vi "svx_Timebase Facade.vi"(0 "Data In":T8, 2 "Display State In":T3={"X Scale"={"Name"="Time", "FString"="%#.2g", "Major Color"=16777238, "Minor Color"=16777216, "Grid Style"=1, "Maximum"=0.5, "Minimum"=0.0, "Autoscale"=TRUE, "Show Scale Label"={"Probe X"=FALSE, "Probe Y"=TRUE}, "Show Scale"={"Probe X"=TRUE, "Probe Y"=TRUE}, "Autoscale Once"=FALSE}, "Y Scale"={"Name"="Amplitude", "FString"="%#.2g", "Major Color"=16777238, "Minor Color"=16777216, "Scale Visible"=TRUE, " Label Visible"=TRUE, "Grid Style"=1, "Autoscale"=TRUE, "Maximum"={"Probe X"=1.0, "Probe Y"=1.0}, "Minimum"={"Probe X"=-1.0, "Probe Y"=-1.0}, "Autoscale Once"=FALSE}, "Plot"={"Point Style"=0, "Line Width"=0, "Line Style"=0, "Plot Color"=16860, "Point/fill"=16860}, "Tacho Point Color"=16711680, "Property Name"=[], "Container Bounds"={"Width"=640, "Height"=360}, "Background color"=16777226, "Legend Visible"=TRUE, "Scale Range Change"=refnum, "Strings[]"={"Custom pair name"=FALSE, "Row Strings []"=[], "Column Strings []"=[]}, "Cursor"={"Cursor Point Style"=13, "Cursor Style"=5, "Cursor Line Width"=1, "Cursor Line Style"=0, "Cursor Color"=16860, "Cursor Name Visible"=TRUE, "Cursor Visible"=TRUE, "Cursor Lock"=FALSE, "Cursor Index"=0}, "Index"=[], "Legend Width"=200, " Parents Tags"=[], "Children Tags"=[], "Open?"=[], "Label"="Timebase Plot", "Cursor X Pos"={"X"=0.0, "Y"=0.0}, "Cursor Y Pos"={"X"=0.0, "Y"=0.0}, "Graph Type"=enum."Probe X and Y", "Prev Graph Type"=enum."Probe X and Y", "Prev Legend Visible"=TRUE, "Cursor Release"=refnum, "Pair Strings Changed?"=FALSE, "Cursor ID"=refnum, "Legend Background"=16777226, "Legend Font"=16777222, "Probe Y Label"="Probe Y", "Probe X Label"="Probe X", "Probe X Label Visible"=TRUE, "Probe Y Label Visible"=TRUE, "Tree Item Width"=200, "# Custom RowStr"=0, "# Custom ColStr"=0, "Property Name"=refnum, "Data Related State"=refnum}, 3 "Container State":T7) -> (6 "Data Out":T8, 7 "Display State Out":T3={"X Scale"={"Name"="Time", "FString"="%#.2g", "Major Color"=16777238, "Minor Color"=16777216, "Grid Style"=1, "Maximum"=0.5, "Minimum"=0.0, "Autoscale"=TRUE, "Show Scale Label"={"Probe X"=FALSE, "Probe Y"=TRUE}, "Show Scale"={"Probe X"=TRUE, "Probe Y"=TRUE}, "Autoscale Once"=FALSE}, "Y Scale"={"Name"="Amplitude", "FString"="%#.2g", "Major Color"=16777238, "Minor Color"=16777216, "Scale Visible"=TRUE, " Label Visible"=TRUE, "Grid Style"=1, "Autoscale"=TRUE, "Maximum"={"Probe X"=1.0, "Probe Y"=1.0}, "Minimum"={"Probe X"=-1.0, "Probe Y"=-1.0}, "Autoscale Once"=FALSE}, "Plot"={"Point Style"=0, "Line Width"=0, "Line Style"=0, "Plot Color"=16860, "Point/fill"=16860}, "Tacho Point Color"=16711680, "Property Name"=[], "Container Bounds"={"Width"=640, "Height"=360}, "Background color"=16777226, "Legend Visible"=TRUE, "Scale Range Change"=refnum, "Strings[]"={"Custom pair name"=FALSE, "Row Strings []"=[], "Column Strings []"=[]}, "Cursor"={"Cursor Point Style"=13, "Cursor Style"=5, "Cursor Line Width"=1, "Cursor Line Style"=0, "Cursor Color"=16860, "Cursor Name Visible"=TRUE, "Cursor Visible"=TRUE, "Cursor Lock"=FALSE, "Cursor Index"=0}, "Index"=[], "Legend Width"=200, " Parents Tags"=[], "Children Tags"=[], "Open?"=[], "Label"="Timebase Plot", "Cursor X Pos"={"X"=0.0, "Y"=0.0}, "Cursor Y Pos"={"X"=0.0, "Y"=0.0}, "Graph Type"=enum."Probe X and Y", "Prev Graph Type"=enum."Probe X and Y", "Prev Legend Visible"=TRUE, "Cursor Release"=refnum, "Pair Strings Changed?"=FALSE, "Cursor ID"=refnum, "Legend Background"=16777226, "Legend Font"=16777222, "Probe Y Label"="Probe Y", "Probe X Label"="Probe X", "Probe X Label Visible"=TRUE, "Probe Y Label Visible"=TRUE, "Tree Item Width"=200, "# Custom RowStr"=0, "# Custom ColStr"=0, "Property Name"=refnum, "Data Related State"=refnum}, 8 "Action":T2)   [LabVIEW 2017, in "SVX Timebase.xctl"]
uses:
  <vilib>/addons/_XControls/Timebase Plot/SVX Timebase.xctl
  <vilib>/addons/_XControls/Timebase Plot/subVIs/svx_Timebase Data.ctl
  <vilib>/_xctls/Container State.ctl
  <vilib>/addons/_XControls/Timebase Plot/subVIs/svx_Timebase State.ctl
  <vilib>/addons/_XControls/Timebase Plot/subVIs/svx_Timebase Bounds.ctl
  <vilib>/addons/_XControls/Timebase Plot/subVIs/svx_Timebase Graph Types.ctl
  <vilib>/addons/_XControls/Timebase Plot/subVIs/svx_Timebase Data Related State.ctl
  <vilib>/_xctls/Action.ctl
  <vilib>/Utility/miscctls.llb/LVPoint32TypeDef.ctl
  <vilib>/addons/_XControls/Timebase Plot/subVIs/svx_Timebase Core States.ctl
  <vilib>/Utility/cursorutil.llb/Set Cursor (Icon Pict).vi
  <vilib>/Utility/cursorutil.llb/Set Cursor (Cursor ID).vi
  <vilib>/_xctls/XControlSupport.lvlib
panel:
  out "Coords":T1
  out "Orig Legend Width":u32
  out "Orig Coord":i32
  in  "Split":bool
  out "cursor X info":string
  out "cursor Y info":string
  out "Probe Y":T9(graph)=[{"orbit plot X"=[1.0], "orbit plot Y"=[2.0]}, {"orbit plot X"=[2.0], "orbit plot Y"=[4.0]}]
  out "Probe X":T9(graph)=[{"orbit plot X"=[1.0], "orbit plot Y"=[2.0]}, {"orbit plot X"=[2.0], "orbit plot Y"=[4.0]}]
  in  "Tree":string(tree)="Order 3.00"
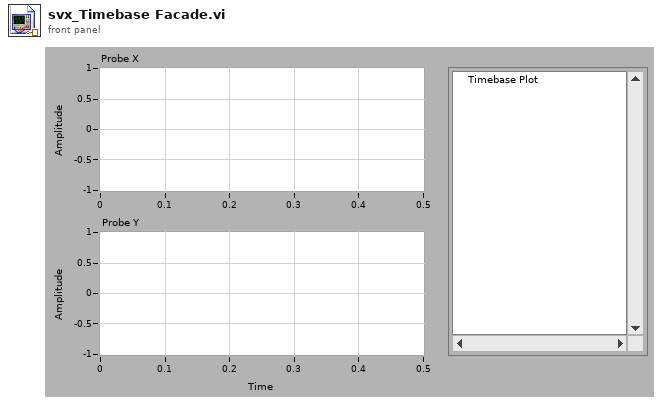
[diagram p1: front panel]
types:
  T1 = typedef "LVPoint32TypeDef.ctl" = cluster{"Horizontal":i32, "Vertical":i32}
  T2 = typedef "XControlSupport.lvlib/Action.ctl" = cluster{"Data Changed?":bool, "State Changed?":bool, "Action Name":string}
  T3 = typedef "SVX Timebase.xctl/svx_Timebase State.ctl" = cluster{"X Scale":cluster{"Name":string, "FString":string, "Major Color":u32, "Minor Color":u32, "Grid Style":u16, "Maximum":dbl, "Minimum":dbl, "Autoscale":bool, "Show Scale Label":cluster{"Probe X":bool, "Probe Y":bool}, "Show Scale":cluster{"Probe X":bool, "Probe Y":bool}, "Autoscale Once":bool}, "Y Scale":cluster{"Name":string, "FString":string, "Major Color":u32, "Minor Color":u32, "Scale Visible":bool, " Label Visible":bool, "Grid Style":u16, "Autoscale":bool, "Maximum":cluster{"Probe X":dbl, "Probe Y":dbl}, "Minimum":cluster{"Probe X":dbl, "Probe Y":dbl}, "Autoscale Once":bool}, "Plot":cluster{"Point Style":u8, "Line Width":u8, "Line Style":u8, "Plot Color":u32, "Point/fill":u32}, "Tacho Point Color":u32, "Property Name":string[], "Container Bounds":T4, "Background color":u32, "Legend Visible":bool, "Scale Range Change":refnum<user-event>, "Strings[]":cluster{"Custom pair name":bool, "Row Strings []":string[], "Column Strings []":string[]}, "Cursor":cluster{"Cursor Point Style":u8, "Cursor Style":u8, "Cursor Line Width":u8, "Cursor Line Style":u8, "Cursor Color":u32, "Cursor Name Visible":bool, "Cursor Visible":bool, "Cursor Lock":bool, "Cursor Index":i32}, "Index":cluster{"Pair Index":u32, "Order Index":u32}[], "Legend Width":u32, " Parents Tags":string[], "Children Tags":string[], "Open?":bool[], "Label":string, "Cursor X Pos":cluster{"X":dbl, "Y":dbl}, "Cursor Y Pos":cluster{"X":dbl, "Y":dbl}, "Graph Type":T5, "Prev Graph Type":T5, "Prev Legend Visible":bool, "Cursor Release":refnum<user-event>, "Pair Strings Changed?":bool, "Cursor ID":refnum<k1>, "Legend Background":u32, "Legend Font":u32, "Probe Y Label":string, "Probe X Label":string, "Probe X Label Visible":bool, "Probe Y Label Visible":bool, "Tree Item Width":u32, "# Custom RowStr":u32, "# Custom ColStr":u32, "Property Name":refnum<queue>, "Data Related State":T6}
  T4 = typedef "SVX Timebase.xctl/svx_Timebase Bounds.ctl" = cluster{"Width":u32, "Height":u32}
  T5 = typedef "SVX Timebase.xctl/svx_Timebase Graph Types.ctl" = enum16{"Probe X", "Probe Y", "Probe X and Y"}
  T6 = typedef "SVX Timebase.xctl/svx_Timebase Data Related State.ctl" = refnum<queue>
  T7 = typedef "XControlSupport.lvlib/Container State.ctl" = cluster{"Indicator?":bool, "Run Mode?":bool, " Refnum":refnum<vi>}
  T8 = typedef "SVX Timebase.xctl/svx_Timebase Data.ctl" = cluster{"X":dbl[], "Y":dbl[], "reference":dbl[], "plot type":enum16{"Filtered Plot", "Unfiltered Plot"}, "attribute":variant}[][]
  T9 = cluster{"orbit plot X":dbl[], "orbit plot Y":dbl[]}[]
  T10 = cluster{"PointIdx":i32, "Position":cluster{"Probe X":dbl, "Probe Y":dbl, "Reference":dbl}}
  T11 = cluster{"Minimum":dbl, "Maximum":dbl, "Kind":enum16{"X-Scale", "Y-Scale", "Z-Scale"}, "Graph Type":T5}
  T12 = typedef "SVX Timebase.xctl/svx_Timebase Core States.ctl" = enum16{"None", "[Axis] Range X Scale", "[Axis] Range Y Scale", "[Layout] Graph Type Change", "[Plot] Tacho Point", "[Plot] Grid and BG", "[Cursor] Cursor Info", "[Legend] Pair Strings", "[Data] Plot Data", "[Legend] Checkbox", "[Layout] Update", "[Legend] Tree Open", "[Layout] Legend Visible Change", "[Plot] Data Point", "[Cursor] Appearance", "[Cursor] Index", "[Legend] Color", "[Axis] Axis and Label", "[Axis] Format String", "[Layout] Min Pane Size", "[Data] Index", "[Plot] Caption", "[Data] Legend Strings"}
  T13 = cluster{"Queue Newer?":bool, "State Newer?":bool, "Maximum":dbl, "Minimum":dbl, "Maximum":cluster{"Probe X":dbl, "Probe Y":dbl}, "Minimum":cluster{"Probe X":dbl, "Probe Y":dbl}, "Cursor Index":i32, "Cursor X Pos":cluster{"X":dbl, "Y":dbl}, "Cursor Y Pos":cluster{"X":dbl, "Y":dbl}, "Strings[]":cluster{"Custom pair name":bool, "Row Strings []":string[], "Column Strings []":string[]}, "Index":cluster{"Pair Index":u32, "Order Index":u32}[], "Tree Item Width":u32, "Parents Tags":string[], "Children Tags":string[], "Open?":bool[], "Tree Visible?":bool, "Graph Type":T5, "Container Bounds":T4, "Label":string}
  T14 = cluster{"Custom pair name":bool, "Row Strings []":string[], "Column Strings []":string[]}
  T15 = cluster{"X":dbl[], "Y":dbl[], "reference":dbl[], "plot type":enum16{"Filtered Plot", "Unfiltered Plot"}, "attribute":variant}
  T16 = cluster{"Probe X":refnum<vi>, "Probe Y":refnum<vi>, "Tree":refnum<vi>, "Split":refnum<vi>, "cursor X info":refnum<vi>, "cursor Y info":refnum<vi>}
  T17 = cluster{"Background color":u32, "Major Color":u32, "Minor Color":u32, "Major Color":u32, "Minor Color":u32}
  T18 = cluster{"BG Color":u32, "XScale.MajGrdColor":u32, "XScale.MnrGrdColor":u32, "YScale.MajGrdColor":u32, "YScale.MnrGrdColor":u32}
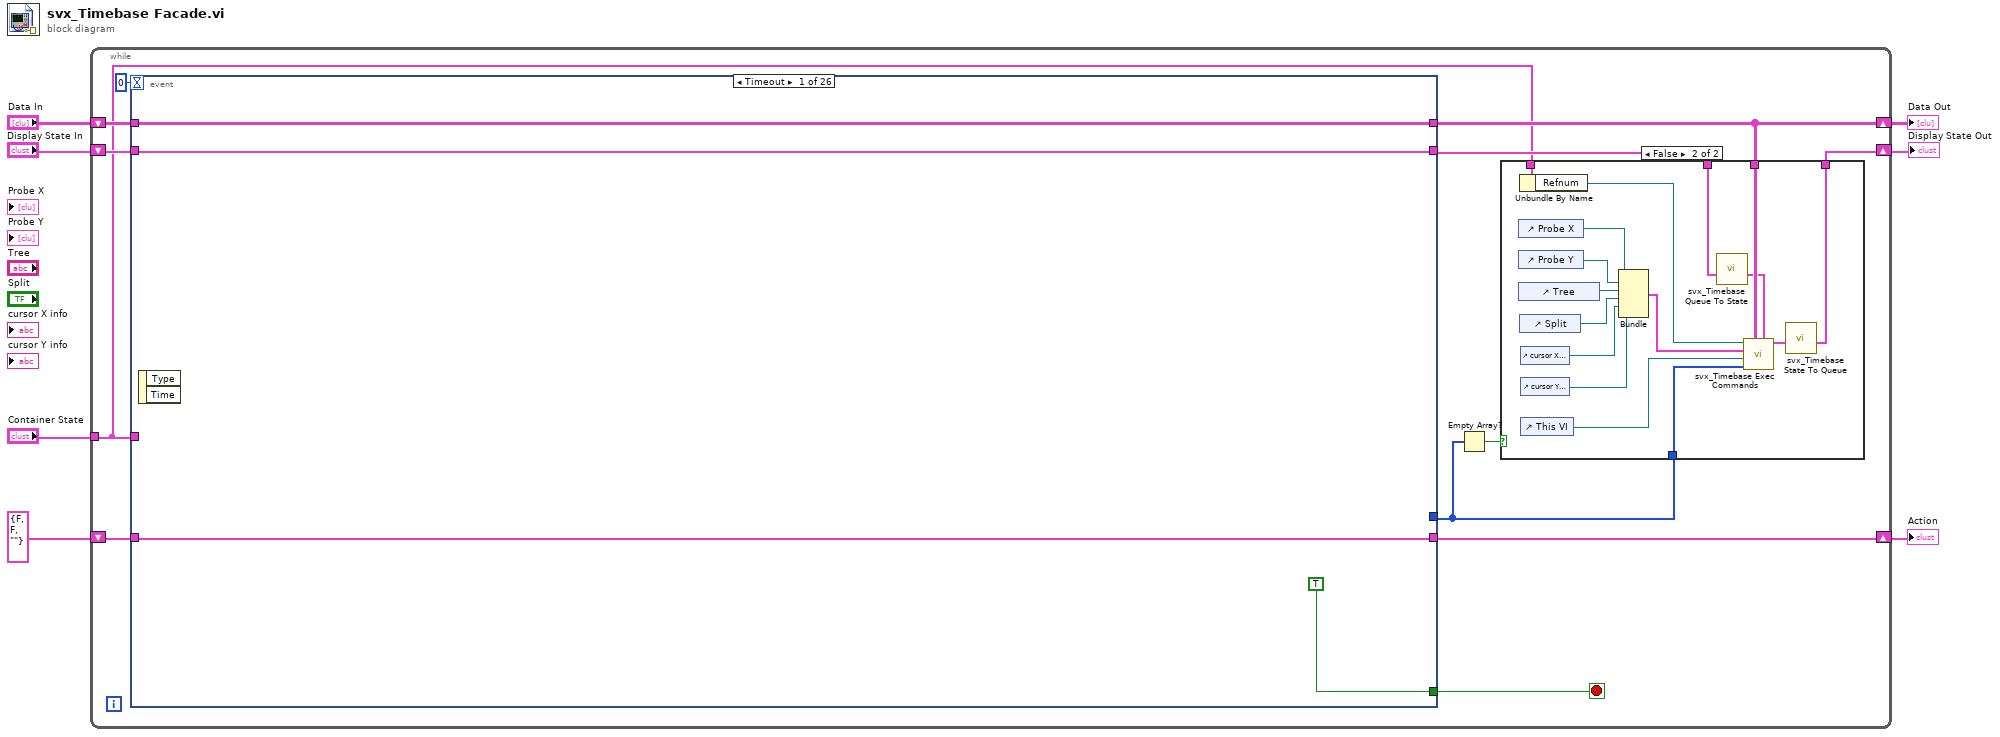
[diagram p0: block diagram]
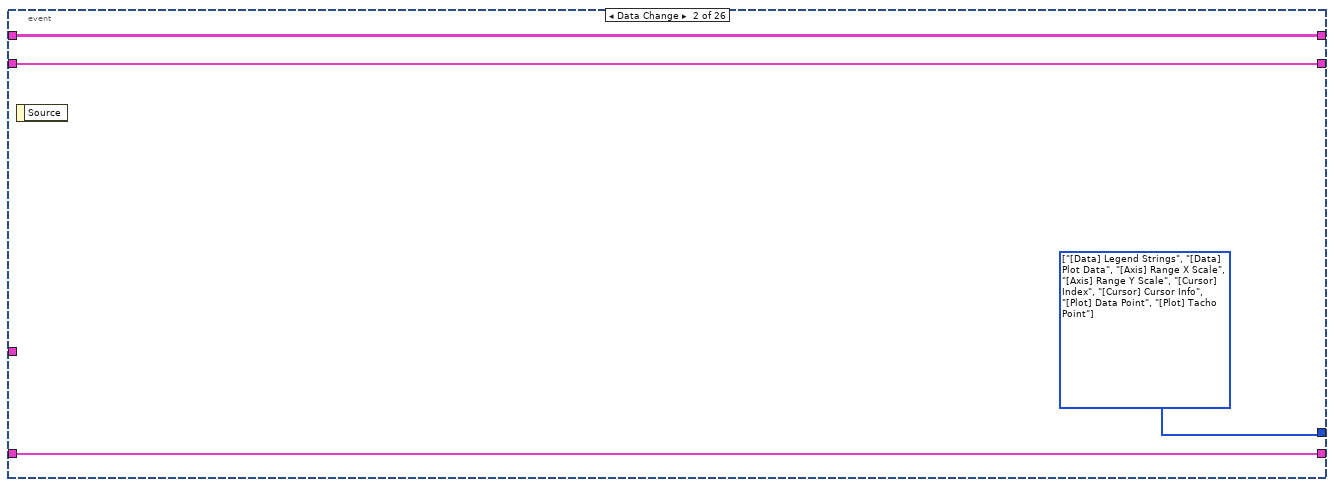
[diagram p3: hidden frame]
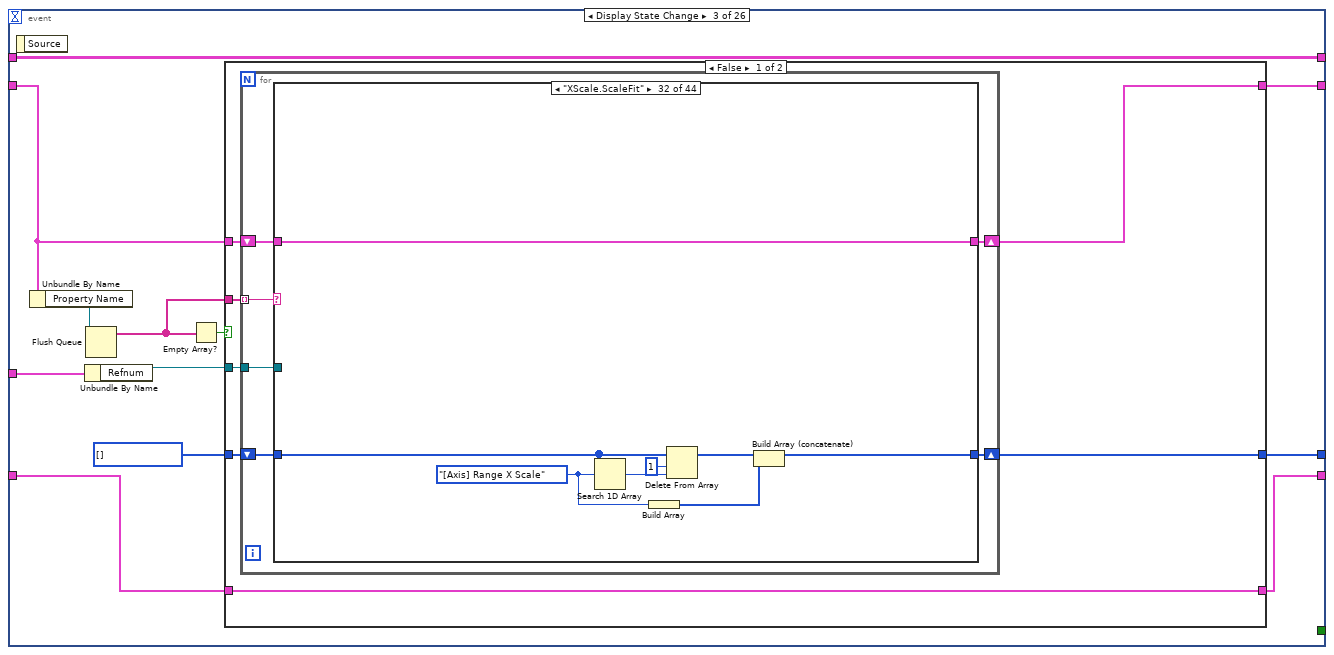
[diagram p4: hidden frame]
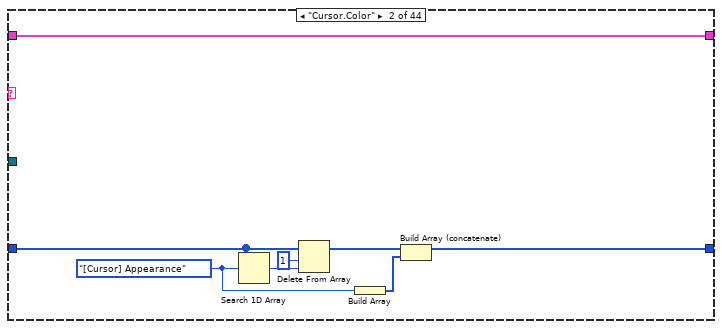
[diagram p6: hidden frame]
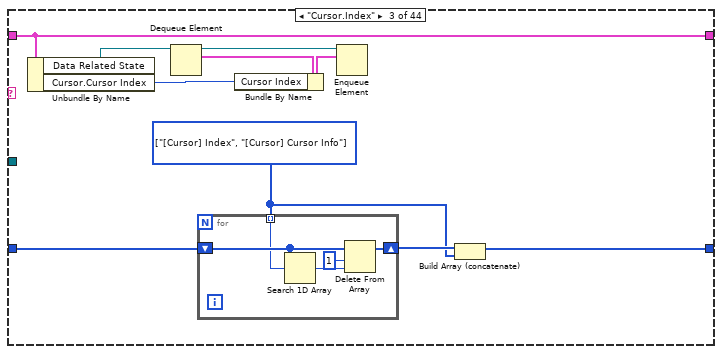
[diagram p7: hidden frame]
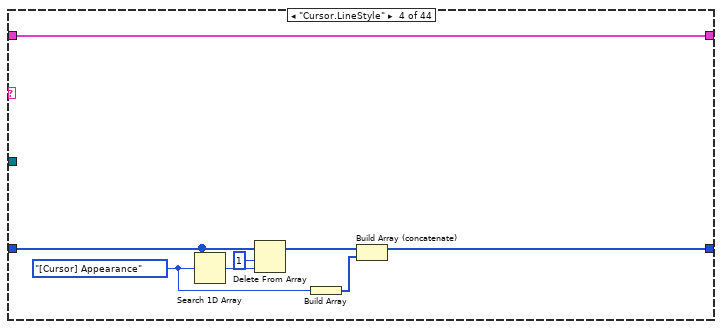
[diagram p8: hidden frame]
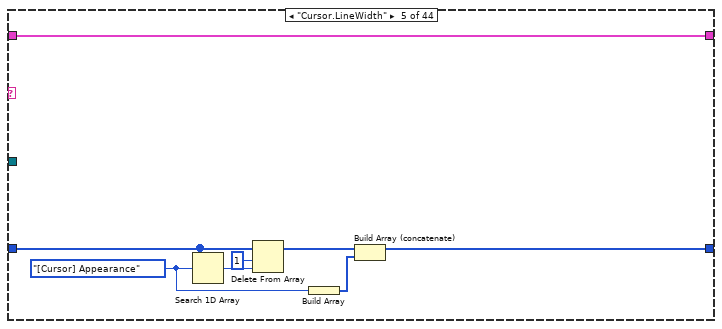
[diagram p9: hidden frame]
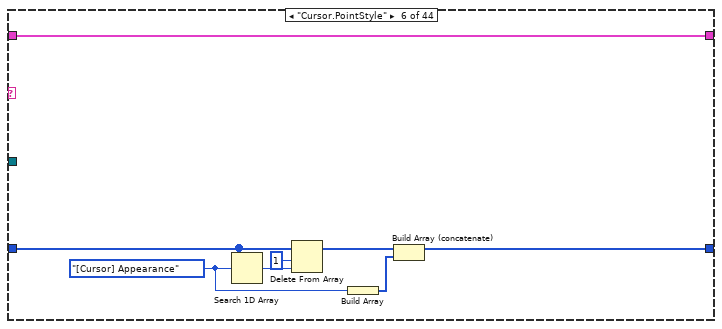
[diagram p10: hidden frame]
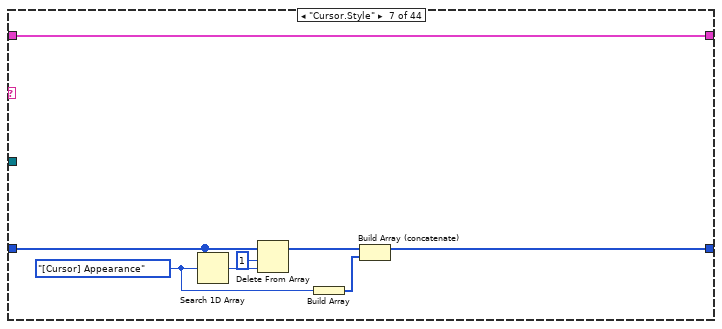
[diagram p11: hidden frame]
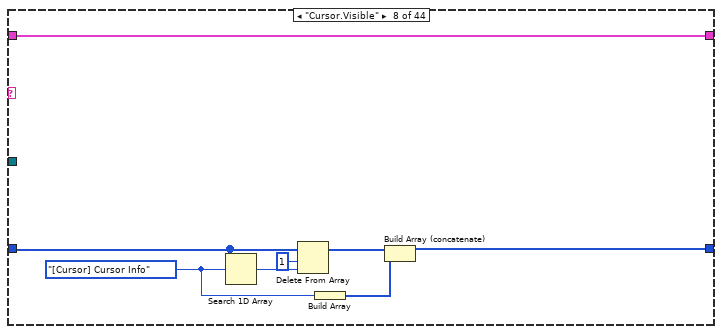
[diagram p12: hidden frame]
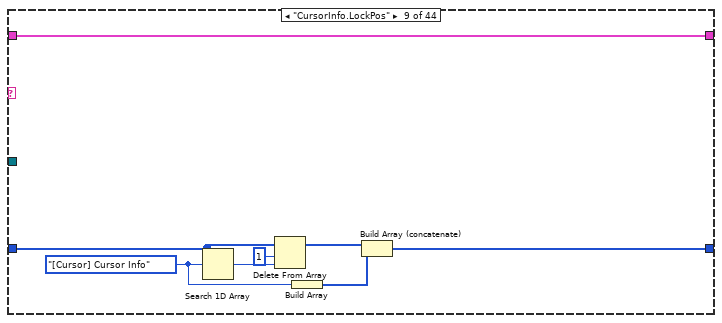
[diagram p13: hidden frame]
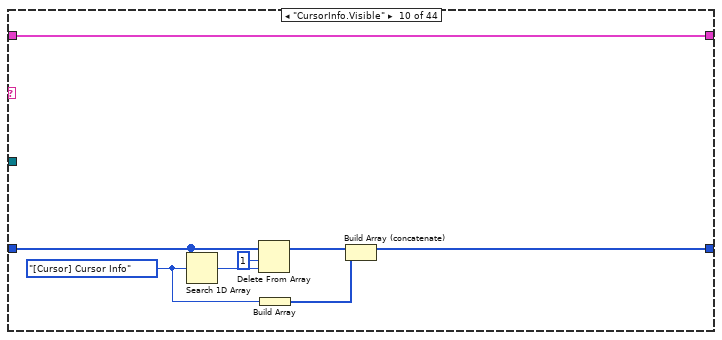
[diagram p14: hidden frame]
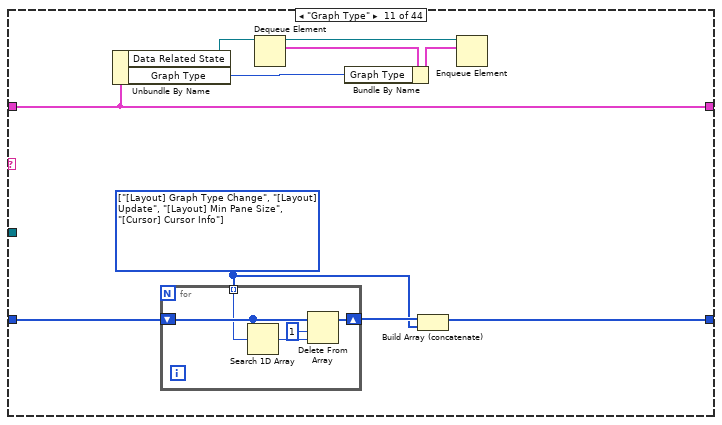
[diagram p15: hidden frame]
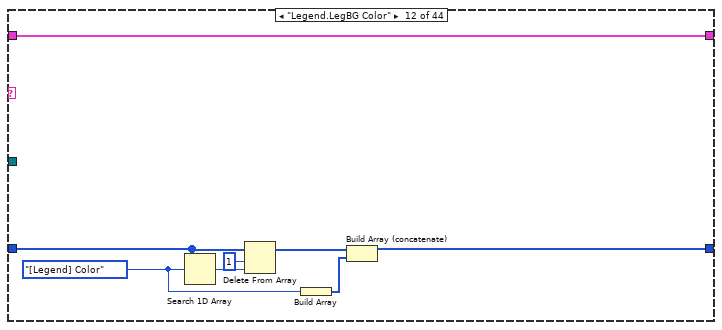
[diagram p16: hidden frame]
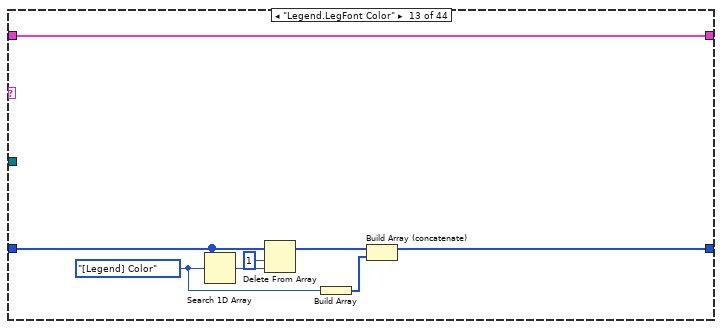
[diagram p17: hidden frame]
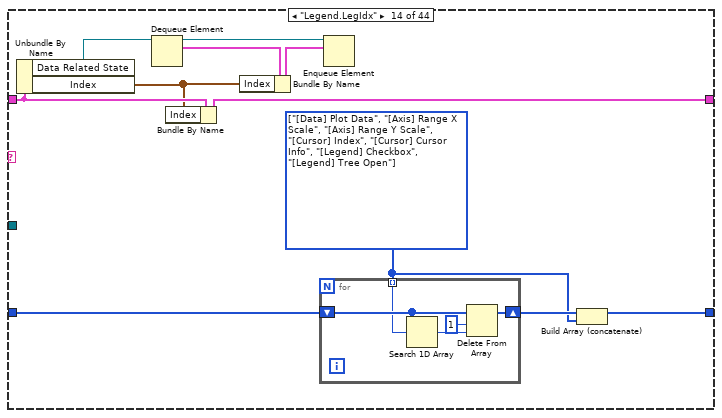
[diagram p18: hidden frame]
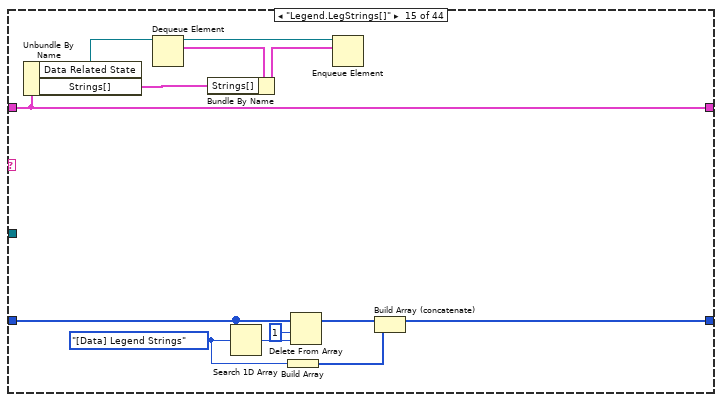
[diagram p19: hidden frame]
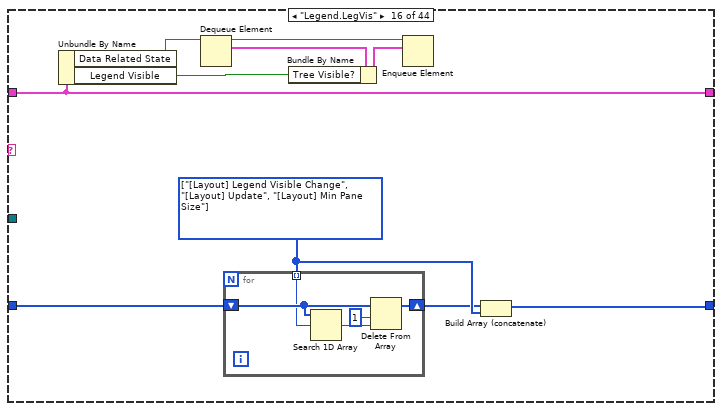
[diagram p20: hidden frame]
diagram:
  n1 = while {
    shift-right: [w12] -> w4
    shift-left: "Display State In" -> [w19]
    tunnel: "Container State" -> [w8]
    shift-right: [w13] -> w7
    shift-left: "Data In" -> [w16]
    shift-right: [w11] -> w2
    shift-left: T2 {"Data Changed?"=FALSE, "State Changed?"=FALSE, "Action Name"=""} ("Action") -> [w15]
    stop <- w18 stop-if-true
    n2 = event shown="[0] Timeout" {
      selector: _ -> [_ _ _ _ _ _ _ _ _ _ _ _ _ _ _ _ _ _ _ _ _ _ _ _ _ _]
      dyn-events: _ -> [_ _ _ _ _ _ _ _ _ _ _ _ _ _ _ _ _ _ _ _ _ _ _ _ _ _]
      timeout: 0 -> [_ _ _ _ _ _ _ _ _ _ _ _ _ _ _ _ _ _ _ _ _ _ _ _ _ _]
      tunnel: w19 -> [w38 w43 w45 w490 w493 w494 w510 w538 w565 w609 w654 w660 w665 w695 w851 w860 w945 w973 w1010 w1019 w1025 w1070 w1093 w1114 w1134 w1143]
      tunnel: [w38 w43 w55 w490 w493 w494 w510 w538 w576 w620 w654 w660 w664 w694 w851 w858 w945 w972 w1010 w1019 w1025 w1067 w1090 w1113 w1134 w1143] -> w14
      tunnel: [TRUE _ _ _ _ _ _ _ _ _ _ _ _ _ _ _ _ _ _ _ _ _ _ _ _ _] -> w18
      tunnel: w8 -> [_ _ w52 _ _ _ _ _ _ _ _ w662 _ w690 _ _ _ _ w1014 _ w1022 w1064 w1087 w1108 w1138 _]
      tunnel: w16 -> [w37 w44 w54 w489 w492 w507 w534 w556 w577 w621 w653 w659 w670 w693 w850 w857 w950 w974 w1012 w1020 w1024 w1069 w1092 w1116 w1135 w1144]
      tunnel: [w37 w44 w54 w489 w492 w507 w534 w556 w577 w621 w653 w659 w669 w693 w850 w857 w950 w974 w1012 w1020 w1024 w1069 w1092 w1116 w1135 w1144] -> w13
      tunnel: [w39 w42 w46 w488 w491 w500 w526 w548 w570 w612 w652 w658 w666 w692 w849 w856 w956 w970 w1011 w1018 w1023 w1065 w1088 w1111 w1133 w1142] -> w11
      tunnel: w15 -> [w39 w42 w47 w488 w491 w500 w527 w548 w571 w613 w652 w658 w667 w691 w849 w859 w957 w971 w1011 w1018 w1023 w1066 w1089 w1112 w1133 w1142]
      tunnel: [_ w41 w48 _ _ w503 w519 w547 w566 w610 _ _ w663 w687 _ w853 w942 w967 _ _ _ w1063 _ w1107 _ _] -> w9
      event Timeout {
        n3 = event-data() -> ()  [unwired: 1 in, 2 out]
      }
      event Data Change {
        w41 = T12[] [enum."[Data] Legend Strings", enum."[Data] Plot Data", enum."[Axis] Range X Scale", enum."[Axis] Range Y Scale", enum."[Cursor] Index", enum."[Cursor] Cursor Info", enum."[Plot] Data Point", enum."[Plot] Tacho Point"] items=["None", "[Axis] Range X Scale", "[Axis] Range Y Scale", "[Layout] Graph Type Change", "[Plot] Tacho Point", "[Plot] Grid and BG", "[Cursor] Cursor Info", "[Legend] Pair Strings", "[Data] Plot Data", "[Legend] Checkbox", "[Layout] Update", "[Legend] Tree Open", "[Layout] Legend Visible Change", "[Plot] Data Point", "[Cursor] Appearance", "[Cursor] Index", "[Legend] Color", "[Axis] Axis and Label", "[Axis] Format String", "[Layout] Min Pane Size", "[Data] Index", "[Plot] Caption", "[Data] Legend Strings"]
        n4 = event-data() -> ()  [unwired: 1 in, 1 out]
      }
      event Display State Change {
        w56 = T12[] [] items=["None", "[Axis] Range X Scale", "[Axis] Range Y Scale", "[Layout] Graph Type Change", "[Plot] Tacho Point", "[Plot] Grid and BG", "[Cursor] Cursor Info", "[Legend] Pair Strings", "[Data] Plot Data", "[Legend] Checkbox", "[Layout] Update", "[Legend] Tree Open", "[Layout] Legend Visible Change", "[Plot] Data Point", "[Cursor] Appearance", "[Cursor] Index", "[Legend] Color", "[Axis] Axis and Label", "[Axis] Format String", "[Layout] Min Pane Size", "[Data] Index", "[Plot] Caption", "[Data] Legend Strings"]
        n5 = event-data() -> ()  [unwired: 1 in, 1 out]
        n6 = Unbundle By Name(w45) -> ("Property Name"=w53:refnum<queue>)
        n7 = Unbundle By Name(w52) -> ("Refnum"=w51:refnum<vi>)
        n8 = Flush Queue(queue=w53) -> (remaining elements=w50:string[])  [unwired: 1 in, 2 out]
        n9 = Empty Array?(array=w50) -> (empty?=w49:bool)
        n10 = case shown="False" w49 {
          tunnel: [w62 w482] -> w48
          tunnel: w56 -> [w63 _]
          tunnel: [w61 w472] -> w55
          tunnel: w45 -> [w60 w472]
          tunnel: w50 -> [w59 _]
          tunnel: w51 -> [w58 _]
          tunnel: w47 -> [w57 w481]
          tunnel: [w57 w481] -> w46
          frame False {
            n11 = for {
              tunnel: w59 -> [w64] mode=indexing
              shift-right: [w68] -> w62
              shift-left: w63 -> [w69]
              shift-right: [w67] -> w61
              shift-left: w60 -> [w65]
              tunnel: w58 -> [w66]
              n12 = case shown="\"XScale.ScaleFit\"" w64 {
                tunnel: w69 -> [w71 w74 w86 w97 w104 w113 w121 w131 w139 w147 w160 w168 w176 w191 w208 w218 w230 w238 w246 w251 w260 w268 w276 w286 w296 w304 w312 w318 w325 w334 w350 w361 w364 w372 w382 w392 w400 w408 w414 w422 w438 w452 w462 w465]
                tunnel: [w71 w73 w87 w96 w105 w112 w120 w134 w142 w150 w159 w167 w175 w190 w209 w219 w229 w241 w245 w252 w259 w267 w275 w285 w299 w307 w315 w317 w326 w333 w349 w360 w363 w371 w381 w395 w403 w411 w413 w421 w437 w451 w461 w464] -> w68
                tunnel: [w70 w72 w81 w95 w103 w111 w119 w127 w135 w143 w151 w166 w174 w183 w200 w216 w226 w234 w242 w250 w258 w266 w274 w282 w292 w300 w308 w316 w324 w332 w340 w359 w362 w370 w378 w388 w396 w404 w412 w420 w430 w444 w460 w463] -> w67
                tunnel: w66 -> [_ _ _ _ _ _ _ _ _ _ _ _ _ _ _ _ _ _ _ _ _ _ _ _ _ _ _ _ _ _ _ _ _ _ _ _ _ _ _ _ _ _ _ _]
                tunnel: w65 -> [w70 w72 w81 w95 w103 w111 w119 w127 w135 w143 w151 w166 w174 w184 w200 w216 w226 w234 w242 w250 w258 w266 w274 w282 w292 w300 w308 w316 w324 w332 w340 w359 w362 w370 w378 w388 w396 w404 w412 w420 w430 w444 w460 w463]
                frame "", Default {
                }
                frame "Cursor.Color" {
                  w76 = svx_Timebase_Core_States."[Cursor] Appearance" ("Property Page User Events")
                  n13 = Search 1D Array(1D array=w74, element=w76) -> (index of element=w79:i32)  [unwired: 1 in]
                  n14 = Delete From Array(array=w74, length=1, index=w79) -> (array with subset deleted=w77:T12[])  [unwired: 1 out]
                  n15 = Build Array(w76) -> (w75:T12[])
                  n16 = Build Array (concatenate)(w77, w75) -> (w73:T12[])
                }
                frame "Cursor.Index" {
                  w88 = T12[] [enum."[Cursor] Index", enum."[Cursor] Cursor Info"] items=["None", "[Axis] Range X Scale", "[Axis] Range Y Scale", "[Layout] Graph Type Change", "[Plot] Tacho Point", "[Plot] Grid and BG", "[Cursor] Cursor Info", "[Legend] Pair Strings", "[Data] Plot Data", "[Legend] Checkbox", "[Layout] Update", "[Legend] Tree Open", "[Layout] Legend Visible Change", "[Plot] Data Point", "[Cursor] Appearance", "[Cursor] Index", "[Legend] Color", "[Axis] Axis and Label", "[Axis] Format String", "[Layout] Min Pane Size", "[Data] Index", "[Plot] Caption", "[Data] Legend Strings"] ("array")
                  n17 = Unbundle By Name(w81) -> ("Data Related State"=w85:T6, "Cursor.Cursor Index"=w80:i32)
                  n18 = Dequeue Element(queue=w85) -> (queue out=w83:T6, element=w84:T13)  [unwired: 2 in, 2 out]
                  n19 = for {
                    shift-right: [w91] -> w89
                    shift-left: w86 -> [w92]
                    tunnel: w88 -> [w90] mode=indexing
                    n20 = Search 1D Array(1D array=w92, element=w90) -> (index of element=w94:i32)  [unwired: 1 in]
                    n21 = Delete From Array(array=w92, length=1, index=w94) -> (array with subset deleted=w91:T12[])  [unwired: 1 out]
                  }
                  n22 = Bundle By Name(cluster=w84, "Cursor Index"=w80) -> (w82:T13)
                  n23 = Enqueue Element(queue=w83, element=w82) -> ()  [unwired: 2 in, 3 out]
                  n24 = Build Array (concatenate)(w89, w88) -> (w87:T12[])
                }
                frame "Cursor.LineStyle" {
                  w99 = svx_Timebase_Core_States."[Cursor] Appearance" ("Property Page User Events")
                  n25 = Search 1D Array(1D array=w97, element=w99) -> (index of element=w102:i32)  [unwired: 1 in]
                  n26 = Delete From Array(array=w97, length=1, index=w102) -> (array with subset deleted=w100:T12[])  [unwired: 1 out]
                  n27 = Build Array(w99) -> (w98:T12[])
                  n28 = Build Array (concatenate)(w100, w98) -> (w96:T12[])
                }
                frame "Cursor.LineWidth" {
                  w107 = svx_Timebase_Core_States."[Cursor] Appearance" ("Property Page User Events")
                  n29 = Search 1D Array(1D array=w104, element=w107) -> (index of element=w110:i32)  [unwired: 1 in]
                  n30 = Delete From Array(array=w104, length=1, index=w110) -> (array with subset deleted=w108:T12[])  [unwired: 1 out]
                  n31 = Build Array(w107) -> (w106:T12[])
                  n32 = Build Array (concatenate)(w108, w106) -> (w105:T12[])
                }
                frame "Cursor.PointStyle" {
                  w115 = svx_Timebase_Core_States."[Cursor] Appearance" ("Property Page User Events")
                  n33 = Search 1D Array(1D array=w113, element=w115) -> (index of element=w118:i32)  [unwired: 1 in]
                  n34 = Delete From Array(array=w113, length=1, index=w118) -> (array with subset deleted=w116:T12[])  [unwired: 1 out]
                  n35 = Build Array(w115) -> (w114:T12[])
                  n36 = Build Array (concatenate)(w116, w114) -> (w112:T12[])
                }
                frame "Cursor.Style" {
                  w123 = svx_Timebase_Core_States."[Cursor] Appearance" ("Property Page User Events")
                  n37 = Search 1D Array(1D array=w121, element=w123) -> (index of element=w126:i32)  [unwired: 1 in]
                  n38 = Delete From Array(array=w121, length=1, index=w126) -> (array with subset deleted=w124:T12[])  [unwired: 1 out]
                  n39 = Build Array(w123) -> (w122:T12[])
                  n40 = Build Array (concatenate)(w124, w122) -> (w120:T12[])
                }
                frame "Cursor.Visible" {
                  w129 = svx_Timebase_Core_States."[Cursor] Cursor Info" ("Property Page User Events")
                  n41 = Search 1D Array(1D array=w131, element=w129) -> (index of element=w133:i32)  [unwired: 1 in]
                  n42 = Delete From Array(array=w131, length=1, index=w133) -> (array with subset deleted=w130:T12[])  [unwired: 1 out]
                  n43 = Build Array(w129) -> (w128:T12[])
                  n44 = Build Array (concatenate)(w130, w128) -> (w134:T12[])
                }
                frame "CursorInfo.LockPos" {
                  w137 = svx_Timebase_Core_States."[Cursor] Cursor Info" ("Property Page User Events")
                  n45 = Search 1D Array(1D array=w139, element=w137) -> (index of element=w141:i32)  [unwired: 1 in]
                  n46 = Delete From Array(array=w139, length=1, index=w141) -> (array with subset deleted=w138:T12[])  [unwired: 1 out]
                  n47 = Build Array(w137) -> (w136:T12[])
                  n48 = Build Array (concatenate)(w138, w136) -> (w142:T12[])
                }
                frame "CursorInfo.Visible" {
                  w145 = svx_Timebase_Core_States."[Cursor] Cursor Info" ("Property Page User Events")
                  n49 = Search 1D Array(1D array=w147, element=w145) -> (index of element=w149:i32)  [unwired: 1 in]
                  n50 = Delete From Array(array=w147, length=1, index=w149) -> (array with subset deleted=w146:T12[])  [unwired: 1 out]
                  n51 = Build Array(w145) -> (w144:T12[])
                  n52 = Build Array (concatenate)(w146, w144) -> (w150:T12[])
                }
                frame "Graph Type" {
                  w157 = T12[] [enum."[Layout] Graph Type Change", enum."[Layout] Update", enum."[Layout] Min Pane Size", enum."[Cursor] Cursor Info"] items=["None", "[Axis] Range X Scale", "[Axis] Range Y Scale", "[Layout] Graph Type Change", "[Plot] Tacho Point", "[Plot] Grid and BG", "[Cursor] Cursor Info", "[Legend] Pair Strings", "[Data] Plot Data", "[Legend] Checkbox", "[Layout] Update", "[Legend] Tree Open", "[Layout] Legend Visible Change", "[Plot] Data Point", "[Cursor] Appearance", "[Cursor] Index", "[Legend] Color", "[Axis] Axis and Label", "[Axis] Format String", "[Layout] Min Pane Size", "[Data] Index", "[Plot] Caption", "[Data] Legend Strings"] ("array")
                  n53 = Unbundle By Name(w151) -> ("Data Related State"=w156:T6, "Graph Type"=w152:T5)
                  n54 = for {
                    shift-right: [w162] -> w158
                    shift-left: w160 -> [w163]
                    tunnel: w157 -> [w161] mode=indexing
                    n55 = Search 1D Array(1D array=w163, element=w161) -> (index of element=w165:i32)  [unwired: 1 in]
                    n56 = Delete From Array(array=w163, length=1, index=w165) -> (array with subset deleted=w162:T12[])  [unwired: 1 out]
                  }
                  n57 = Dequeue Element(queue=w156) -> (queue out=w154:T6, element=w155:T13)  [unwired: 2 in, 2 out]
                  n58 = Bundle By Name(cluster=w155, "Graph Type"=w152) -> (w153:T13)
                  n59 = Build Array (concatenate)(w158, w157) -> (w159:T12[])
                  n60 = Enqueue Element(queue=w154, element=w153) -> ()  [unwired: 2 in, 3 out]
                }
                frame "Legend.LegBG Color" {
                  w170 = svx_Timebase_Core_States."[Legend] Color" ("Property Page User Events")
                  n61 = Search 1D Array(1D array=w168, element=w170) -> (index of element=w173:i32)  [unwired: 1 in]
                  n62 = Delete From Array(array=w168, length=1, index=w173) -> (array with subset deleted=w171:T12[])  [unwired: 1 out]
                  n63 = Build Array(w170) -> (w169:T12[])
                  n64 = Build Array (concatenate)(w171, w169) -> (w167:T12[])
                }
                frame "Legend.LegFont Color" {
                  w178 = svx_Timebase_Core_States."[Legend] Color" ("Property Page User Events")
                  n65 = Search 1D Array(1D array=w176, element=w178) -> (index of element=w181:i32)  [unwired: 1 in]
                  n66 = Delete From Array(array=w176, length=1, index=w181) -> (array with subset deleted=w179:T12[])  [unwired: 1 out]
                  n67 = Build Array(w178) -> (w177:T12[])
                  n68 = Build Array (concatenate)(w179, w177) -> (w175:T12[])
                }
                frame "Legend.LegIdx" {
                  w189 = T12[] [enum."[Data] Plot Data", enum."[Axis] Range X Scale", enum."[Axis] Range Y Scale", enum."[Cursor] Index", enum."[Cursor] Cursor Info", enum."[Legend] Checkbox", enum."[Legend] Tree Open"] items=["None", "[Axis] Range X Scale", "[Axis] Range Y Scale", "[Layout] Graph Type Change", "[Plot] Tacho Point", "[Plot] Grid and BG", "[Cursor] Cursor Info", "[Legend] Pair Strings", "[Data] Plot Data", "[Legend] Checkbox", "[Layout] Update", "[Legend] Tree Open", "[Layout] Legend Visible Change", "[Plot] Data Point", "[Cursor] Appearance", "[Cursor] Index", "[Legend] Color", "[Axis] Axis and Label", "[Axis] Format String", "[Layout] Min Pane Size", "[Data] Index", "[Plot] Caption", "[Data] Legend Strings"]
                  n69 = Unbundle By Name(w184) -> ("Data Related State"=w185:T6, "Index"=w182:cluster{"Pair Index":u32, "Order Index":u32}[])
                  n70 = Dequeue Element(queue=w185) -> (queue out=w187:T6, element=w188:T13)  [unwired: 2 in, 2 out]
                  n71 = Bundle By Name(cluster=w184, "Index"=w182) -> (w183:T3)
                  n72 = Bundle By Name(cluster=w188, "Index"=w182) -> (w186:T13)
                  n73 = for {
                    shift-right: [w194] -> w192
                    shift-left: w191 -> [w195]
                    tunnel: w189 -> [w193] mode=indexing
                    n74 = Search 1D Array(1D array=w195, element=w193) -> (index of element=w197:i32)  [unwired: 1 in]
                    n75 = Delete From Array(array=w195, length=1, index=w197) -> (array with subset deleted=w194:T12[])  [unwired: 1 out]
                  }
                  n76 = Enqueue Element(queue=w187, element=w186) -> ()  [unwired: 2 in, 3 out]
                  n77 = Build Array (concatenate)(w192, w189) -> (w190:T12[])
                }
                frame "Legend.LegStrings[]" {
                  w205 = svx_Timebase_Core_States."[Data] Legend Strings" ("Property Page User Events")
                  n78 = Unbundle By Name(w200) -> ("Data Related State"=w199:T6, "Strings[]"=w198:T14)
                  n79 = Dequeue Element(queue=w199) -> (queue out=w202:T6, element=w203:T13)  [unwired: 2 in, 2 out]
                  n80 = Bundle By Name(cluster=w203, "Strings[]"=w198) -> (w201:T13)
                  n81 = Search 1D Array(1D array=w208, element=w205) -> (index of element=w207:i32)  [unwired: 1 in]
                  n82 = Build Array(w205) -> (w204:T12[])
                  n83 = Delete From Array(array=w208, length=1, index=w207) -> (array with subset deleted=w210:T12[])  [unwired: 1 out]
                  n84 = Enqueue Element(queue=w202, element=w201) -> ()  [unwired: 2 in, 3 out]
                  n85 = Build Array (concatenate)(w210, w204) -> (w209:T12[])
                }
                frame "Legend.LegVis" {
                  w220 = T12[] [enum."[Layout] Legend Visible Change", enum."[Layout] Update", enum."[Layout] Min Pane Size"] items=["None", "[Axis] Range X Scale", "[Axis] Range Y Scale", "[Layout] Graph Type Change", "[Plot] Tacho Point", "[Plot] Grid and BG", "[Cursor] Cursor Info", "[Legend] Pair Strings", "[Data] Plot Data", "[Legend] Checkbox", "[Layout] Update", "[Legend] Tree Open", "[Layout] Legend Visible Change", "[Plot] Data Point", "[Cursor] Appearance", "[Cursor] Index", "[Legend] Color", "[Axis] Axis and Label", "[Axis] Format String", "[Layout] Min Pane Size", "[Data] Index", "[Plot] Caption", "[Data] Legend Strings"] ("array")
                  n86 = Unbundle By Name(w216) -> ("Data Related State"=w215:T6, "Legend Visible"=w211:bool)
                  n87 = Dequeue Element(queue=w215) -> (queue out=w213:T6, element=w214:T13)  [unwired: 2 in, 2 out]
                  n88 = for {
                    shift-right: [w223] -> w217
                    shift-left: w218 -> [w222]
                    tunnel: w220 -> [w221] mode=indexing
                    n89 = Search 1D Array(1D array=w222, element=w221) -> (index of element=w225:i32)  [unwired: 1 in]
                    n90 = Delete From Array(array=w222, length=1, index=w225) -> (array with subset deleted=w223:T12[])  [unwired: 1 out]
                  }
                  n91 = Bundle By Name(cluster=w214, "Tree Visible?"=w211) -> (w212:T13)
                  n92 = Enqueue Element(queue=w213, element=w212) -> ()  [unwired: 2 in, 3 out]
                  n93 = Build Array (concatenate)(w217, w220) -> (w219:T12[])
                }
                frame "Plot Area.BG Color" {
                  w228 = svx_Timebase_Core_States."[Plot] Grid and BG" ("Property Page User Events")
                  n94 = Search 1D Array(1D array=w230, element=w228) -> (index of element=w233:i32)  [unwired: 1 in]
                  n95 = Build Array(w228) -> (w227:T12[])
                  n96 = Delete From Array(array=w230, length=1, index=w233) -> (array with subset deleted=w231:T12[])  [unwired: 1 out]
                  n97 = Build Array (concatenate)(w231, w227) -> (w229:T12[])
                }
                frame "Plot Area.TrigPointColor" {
                  w236 = svx_Timebase_Core_States."[Plot] Tacho Point" ("Property Page User Events")
                  n98 = Search 1D Array(1D array=w238, element=w236) -> (index of element=w240:i32)  [unwired: 1 in]
                  n99 = Build Array(w236) -> (w235:T12[])
                  n100 = Delete From Array(array=w238, length=1, index=w240) -> (array with subset deleted=w237:T12[])  [unwired: 1 out]
                  n101 = Build Array (concatenate)(w237, w235) -> (w241:T12[])
                }
                frame "Plot.Color" {
                  w244 = svx_Timebase_Core_States."[Plot] Data Point" ("Property Page User Events")
                  n102 = Search 1D Array(1D array=w246, element=w244) -> (index of element=w249:i32)  [unwired: 1 in]
                  n103 = Delete From Array(array=w246, length=1, index=w249) -> (array with subset deleted=w247:T12[])  [unwired: 1 out]
                  n104 = Build Array(w244) -> (w243:T12[])
                  n105 = Build Array (concatenate)(w247, w243) -> (w245:T12[])
                }
                frame "Plot.Fill/PtColor" {
                  w254 = svx_Timebase_Core_States."[Plot] Data Point" ("Property Page User Events")
                  n106 = Search 1D Array(1D array=w251, element=w254) -> (index of element=w257:i32)  [unwired: 1 in]
                  n107 = Delete From Array(array=w251, length=1, index=w257) -> (array with subset deleted=w255:T12[])  [unwired: 1 out]
                  n108 = Build Array(w254) -> (w253:T12[])
                  n109 = Build Array (concatenate)(w255, w253) -> (w252:T12[])
                }
                frame "Plot.LineStyle" {
                  w262 = svx_Timebase_Core_States."[Plot] Data Point" ("Property Page User Events")
                  n110 = Search 1D Array(1D array=w260, element=w262) -> (index of element=w265:i32)  [unwired: 1 in]
                  n111 = Delete From Array(array=w260, length=1, index=w265) -> (array with subset deleted=w263:T12[])  [unwired: 1 out]
                  n112 = Build Array(w262) -> (w261:T12[])
                  n113 = Build Array (concatenate)(w263, w261) -> (w259:T12[])
                }
                frame "Plot.LineWidth" {
                  w270 = svx_Timebase_Core_States."[Plot] Data Point" ("Property Page User Events")
                  n114 = Search 1D Array(1D array=w268, element=w270) -> (index of element=w273:i32)  [unwired: 1 in]
                  n115 = Delete From Array(array=w268, length=1, index=w273) -> (array with subset deleted=w271:T12[])  [unwired: 1 out]
                  n116 = Build Array(w270) -> (w269:T12[])
                  n117 = Build Array (concatenate)(w271, w269) -> (w267:T12[])
                }
                frame "Plot.PointStyle" {
                  w278 = svx_Timebase_Core_States."[Plot] Data Point" ("Property Page User Events")
                  n118 = Search 1D Array(1D array=w276, element=w278) -> (index of element=w281:i32)  [unwired: 1 in]
                  n119 = Build Array(w278) -> (w277:T12[])
                  n120 = Delete From Array(array=w276, length=1, index=w281) -> (array with subset deleted=w279:T12[])  [unwired: 1 out]
                  n121 = Build Array (concatenate)(w279, w277) -> (w275:T12[])
                }
                frame "XScale.FormatString" {
                  w283 = T12[] [enum."[Axis] Format String", enum."[Cursor] Cursor Info"] items=["None", "[Axis] Range X Scale", "[Axis] Range Y Scale", "[Layout] Graph Type Change", "[Plot] Tacho Point", "[Plot] Grid and BG", "[Cursor] Cursor Info", "[Legend] Pair Strings", "[Data] Plot Data", "[Legend] Checkbox", "[Layout] Update", "[Legend] Tree Open", "[Layout] Legend Visible Change", "[Plot] Data Point", "[Cursor] Appearance", "[Cursor] Index", "[Legend] Color", "[Axis] Axis and Label", "[Axis] Format String", "[Layout] Min Pane Size", "[Data] Index", "[Plot] Caption", "[Data] Legend Strings"] ("array")
                  n122 = for {
                    shift-right: [w288] -> w284
                    shift-left: w286 -> [w289]
                    tunnel: w283 -> [w287] mode=indexing
                    n123 = Search 1D Array(1D array=w289, element=w287) -> (index of element=w291:i32)  [unwired: 1 in]
                    n124 = Delete From Array(array=w289, length=1, index=w291) -> (array with subset deleted=w288:T12[])  [unwired: 1 out]
                  }
                  n125 = Build Array (concatenate)(w284, w283) -> (w285:T12[])
                }
                frame "XScale.GridStyle" {
                  w294 = svx_Timebase_Core_States."[Plot] Grid and BG" ("Property Page User Events")
                  n126 = Search 1D Array(1D array=w296, element=w294) -> (index of element=w298:i32)  [unwired: 1 in]
                  n127 = Build Array(w294) -> (w293:T12[])
                  n128 = Delete From Array(array=w296, length=1, index=w298) -> (array with subset deleted=w295:T12[])  [unwired: 1 out]
                  n129 = Build Array (concatenate)(w295, w293) -> (w299:T12[])
                }
                frame "XScale.MajGrdColor" {
                  w302 = svx_Timebase_Core_States."[Plot] Grid and BG" ("Property Page User Events")
                  n130 = Search 1D Array(1D array=w304, element=w302) -> (index of element=w306:i32)  [unwired: 1 in]
                  n131 = Build Array(w302) -> (w301:T12[])
                  n132 = Delete From Array(array=w304, length=1, index=w306) -> (array with subset deleted=w303:T12[])  [unwired: 1 out]
                  n133 = Build Array (concatenate)(w303, w301) -> (w307:T12[])
                }
                frame "XScale.MnrGrdColor" {
                  w310 = svx_Timebase_Core_States."[Plot] Grid and BG" ("Property Page User Events")
                  n134 = Search 1D Array(1D array=w312, element=w310) -> (index of element=w314:i32)  [unwired: 1 in]
                  n135 = Build Array(w310) -> (w309:T12[])
                  n136 = Delete From Array(array=w312, length=1, index=w314) -> (array with subset deleted=w311:T12[])  [unwired: 1 out]
                  n137 = Build Array (concatenate)(w311, w309) -> (w315:T12[])
                }
                frame "XScale.NameLbl.Text" {
                  w320 = svx_Timebase_Core_States."[Axis] Axis and Label" ("Property Page User Events")
                  n138 = Search 1D Array(1D array=w318, element=w320) -> (index of element=w323:i32)  [unwired: 1 in]
                  n139 = Delete From Array(array=w318, length=1, index=w323) -> (array with subset deleted=w321:T12[])  [unwired: 1 out]
                  n140 = Build Array(w320) -> (w319:T12[])
                  n141 = Build Array (concatenate)(w321, w319) -> (w317:T12[])
                }
                frame "XScale.NameLbl.Visible.ProbeX" {
                  w328 = svx_Timebase_Core_States."[Axis] Axis and Label" ("Property Page User Events")
                  n142 = Search 1D Array(1D array=w325, element=w328) -> (index of element=w331:i32)  [unwired: 1 in]
                  n143 = Delete From Array(array=w325, length=1, index=w331) -> (array with subset deleted=w329:T12[])  [unwired: 1 out]
                  n144 = Build Array(w328) -> (w327:T12[])
                  n145 = Build Array (concatenate)(w329, w327) -> (w326:T12[])
                }
                frame "XScale.NameLbl.Visible.ProbeY" {
                  w336 = svx_Timebase_Core_States."[Axis] Axis and Label" ("Property Page User Events")
                  n146 = Search 1D Array(1D array=w334, element=w336) -> (index of element=w339:i32)  [unwired: 1 in]
                  n147 = Delete From Array(array=w334, length=1, index=w339) -> (array with subset deleted=w337:T12[])  [unwired: 1 out]
                  n148 = Build Array(w336) -> (w335:T12[])
                  n149 = Build Array (concatenate)(w337, w335) -> (w333:T12[])
                }
                frame "XScale.Range" {
                  w348 = svx_Timebase_Core_States."[Axis] Range X Scale" ("Property Page User Events")
                  n150 = Unbundle By Name(w340) -> ("Data Related State"=w343:T6, "X Scale.Maximum"=w342:dbl, "X Scale.Minimum"=w341:dbl)
                  n151 = Dequeue Element(queue=w343) -> (queue out=w345:T6, element=w346:T13)  [unwired: 2 in, 2 out]
                  n152 = Bundle By Name(cluster=w346, "Maximum"=w342, "Minimum"=w341) -> (w344:T13)
                  n153 = Search 1D Array(1D array=w350, element=w348) -> (index of element=w353:i32)  [unwired: 1 in]
                  n154 = Build Array(w348) -> (w347:T12[])
                  n155 = Delete From Array(array=w350, length=1, index=w353) -> (array with subset deleted=w351:T12[])  [unwired: 1 out]
                  n156 = Enqueue Element(queue=w345, element=w344) -> ()  [unwired: 2 in, 3 out]
                  n157 = Build Array (concatenate)(w351, w347) -> (w349:T12[])
                }
                frame "XScale.ScaleFit" {
                  w355 = svx_Timebase_Core_States."[Axis] Range X Scale" ("Property Page User Events")
                  n158 = Search 1D Array(1D array=w361, element=w355) -> (index of element=w358:i32)  [unwired: 1 in]
                  n159 = Build Array(w355) -> (w354:T12[])
                  n160 = Delete From Array(array=w361, length=1, index=w358) -> (array with subset deleted=w356:T12[])  [unwired: 1 out]
                  n161 = Build Array (concatenate)(w356, w354) -> (w360:T12[])
                }
                frame "XScale.Visible.ProbeX" {
                  w366 = svx_Timebase_Core_States."[Axis] Axis and Label" ("Property Page User Events")
                  n162 = Search 1D Array(1D array=w364, element=w366) -> (index of element=w369:i32)  [unwired: 1 in]
                  n163 = Delete From Array(array=w364, length=1, index=w369) -> (array with subset deleted=w367:T12[])  [unwired: 1 out]
                  n164 = Build Array(w366) -> (w365:T12[])
                  n165 = Build Array (concatenate)(w367, w365) -> (w363:T12[])
                }
                frame "XScale.Visible.ProbeY" {
                  w374 = svx_Timebase_Core_States."[Axis] Axis and Label" ("Property Page User Events")
                  n166 = Search 1D Array(1D array=w372, element=w374) -> (index of element=w377:i32)  [unwired: 1 in]
                  n167 = Delete From Array(array=w372, length=1, index=w377) -> (array with subset deleted=w375:T12[])  [unwired: 1 out]
                  n168 = Build Array(w374) -> (w373:T12[])
                  n169 = Build Array (concatenate)(w375, w373) -> (w371:T12[])
                }
                frame "YScale.FormatString" {
                  w379 = T12[] [enum."[Axis] Format String", enum."[Cursor] Cursor Info"] items=["None", "[Axis] Range X Scale", "[Axis] Range Y Scale", "[Layout] Graph Type Change", "[Plot] Tacho Point", "[Plot] Grid and BG", "[Cursor] Cursor Info", "[Legend] Pair Strings", "[Data] Plot Data", "[Legend] Checkbox", "[Layout] Update", "[Legend] Tree Open", "[Layout] Legend Visible Change", "[Plot] Data Point", "[Cursor] Appearance", "[Cursor] Index", "[Legend] Color", "[Axis] Axis and Label", "[Axis] Format String", "[Layout] Min Pane Size", "[Data] Index", "[Plot] Caption", "[Data] Legend Strings"] ("array")
                  n170 = for {
                    shift-right: [w384] -> w380
                    shift-left: w382 -> [w385]
                    tunnel: w379 -> [w383] mode=indexing
                    n171 = Search 1D Array(1D array=w385, element=w383) -> (index of element=w387:i32)  [unwired: 1 in]
                    n172 = Delete From Array(array=w385, length=1, index=w387) -> (array with subset deleted=w384:T12[])  [unwired: 1 out]
                  }
                  n173 = Build Array (concatenate)(w380, w379) -> (w381:T12[])
                }
                frame "YScale.GridStyle" {
                  w390 = svx_Timebase_Core_States."[Plot] Grid and BG" ("Property Page User Events")
                  n174 = Search 1D Array(1D array=w392, element=w390) -> (index of element=w394:i32)  [unwired: 1 in]
                  n175 = Build Array(w390) -> (w389:T12[])
                  n176 = Delete From Array(array=w392, length=1, index=w394) -> (array with subset deleted=w391:T12[])  [unwired: 1 out]
                  n177 = Build Array (concatenate)(w391, w389) -> (w395:T12[])
                }
                frame "YScale.MajGrdColor" {
                  w398 = svx_Timebase_Core_States."[Plot] Grid and BG" ("Property Page User Events")
                  n178 = Search 1D Array(1D array=w400, element=w398) -> (index of element=w402:i32)  [unwired: 1 in]
                  n179 = Build Array(w398) -> (w397:T12[])
                  n180 = Delete From Array(array=w400, length=1, index=w402) -> (array with subset deleted=w399:T12[])  [unwired: 1 out]
                  n181 = Build Array (concatenate)(w399, w397) -> (w403:T12[])
                }
                frame "YScale.MnrGrdColor" {
                  w406 = svx_Timebase_Core_States."[Plot] Grid and BG" ("Property Page User Events")
                  n182 = Search 1D Array(1D array=w408, element=w406) -> (index of element=w410:i32)  [unwired: 1 in]
                  n183 = Build Array(w406) -> (w405:T12[])
                  n184 = Delete From Array(array=w408, length=1, index=w410) -> (array with subset deleted=w407:T12[])  [unwired: 1 out]
                  n185 = Build Array (concatenate)(w407, w405) -> (w411:T12[])
                }
                frame "YScale.NameLbl.Text" {
                  w416 = svx_Timebase_Core_States."[Axis] Axis and Label" ("Property Page User Events")
                  n186 = Search 1D Array(1D array=w414, element=w416) -> (index of element=w419:i32)  [unwired: 1 in]
                  n187 = Delete From Array(array=w414, length=1, index=w419) -> (array with subset deleted=w417:T12[])  [unwired: 1 out]
                  n188 = Build Array(w416) -> (w415:T12[])
                  n189 = Build Array (concatenate)(w417, w415) -> (w413:T12[])
                }
                frame "YScale.NameLbl.Visible" {
                  w424 = svx_Timebase_Core_States."[Axis] Axis and Label" ("Property Page User Events")
                  n190 = Search 1D Array(1D array=w422, element=w424) -> (index of element=w427:i32)  [unwired: 1 in]
                  n191 = Delete From Array(array=w422, length=1, index=w427) -> (array with subset deleted=w425:T12[])  [unwired: 1 out]
                  n192 = Build Array(w424) -> (w423:T12[])
                  n193 = Build Array (concatenate)(w425, w423) -> (w421:T12[])
                }
                frame "YScale.Range.ProbeX" {
                  w436 = svx_Timebase_Core_States."[Axis] Range Y Scale" ("Property Page User Events")
                  n194 = Unbundle By Name(w430) -> ("Data Related State"=w431:T6, "Y Scale.Maximum.Probe X"=w429:dbl, "Y Scale.Minimum.Probe X"=w428:dbl)
                  n195 = Dequeue Element(queue=w431) -> (queue out=w433:T6, element=w434:T13)  [unwired: 2 in, 2 out]
                  n196 = Bundle By Name(cluster=w434, "Maximum.Probe X"=w429, "Minimum.Probe X"=w428) -> (w432:T13)
                  n197 = Search 1D Array(1D array=w438, element=w436) -> (index of element=w441:i32)  [unwired: 1 in]
                  n198 = Enqueue Element(queue=w433, element=w432) -> ()  [unwired: 2 in, 3 out]
                  n199 = Delete From Array(array=w438, length=1, index=w441) -> (array with subset deleted=w439:T12[])  [unwired: 1 out]
                  n200 = Build Array(w436) -> (w435:T12[])
                  n201 = Build Array (concatenate)(w439, w435) -> (w437:T12[])
                }
                frame "YScale.Range.ProbeY" {
                  w450 = svx_Timebase_Core_States."[Axis] Range Y Scale" ("Property Page User Events")
                  n202 = Unbundle By Name(w444) -> ("Data Related State"=w445:T6, "Y Scale.Maximum.Probe Y"=w443:dbl, "Y Scale.Minimum.Probe Y"=w442:dbl)
                  n203 = Dequeue Element(queue=w445) -> (queue out=w447:T6, element=w448:T13)  [unwired: 2 in, 2 out]
                  n204 = Bundle By Name(cluster=w448, "Maximum.Probe Y"=w443, "Minimum.Probe Y"=w442) -> (w446:T13)
                  n205 = Search 1D Array(1D array=w452, element=w450) -> (index of element=w455:i32)  [unwired: 1 in]
                  n206 = Delete From Array(array=w452, length=1, index=w455) -> (array with subset deleted=w453:T12[])  [unwired: 1 out]
                  n207 = Build Array(w450) -> (w449:T12[])
                  n208 = Enqueue Element(queue=w447, element=w446) -> ()  [unwired: 2 in, 3 out]
                  n209 = Build Array (concatenate)(w453, w449) -> (w451:T12[])
                }
                frame "YScale.ScaleFit" {
                  w456 = svx_Timebase_Core_States."[Axis] Range Y Scale" ("Property Page User Events")
                  n210 = Search 1D Array(1D array=w462, element=w456) -> (index of element=w459:i32)  [unwired: 1 in]
                  n211 = Delete From Array(array=w462, length=1, index=w459) -> (array with subset deleted=w457:T12[])  [unwired: 1 out]
                  n212 = Build Array (concatenate)(w457, w456) -> (w461:T12[])
                }
                frame "YScale.Visible" {
                  w467 = svx_Timebase_Core_States."[Axis] Axis and Label" ("Property Page User Events")
                  n213 = Search 1D Array(1D array=w465, element=w467) -> (index of element=w470:i32)  [unwired: 1 in]
                  n214 = Delete From Array(array=w465, length=1, index=w470) -> (array with subset deleted=w468:T12[])  [unwired: 1 out]
                  n215 = Build Array(w467) -> (w466:T12[])
                  n216 = Build Array (concatenate)(w468, w466) -> (w464:T12[])
                }
              }
            }
          }
          frame True {
            w482 = T12[] [enum."[Data] Legend Strings", enum."[Data] Plot Data", enum."[Plot] Data Point", enum."[Plot] Tacho Point", enum."[Plot] Caption", enum."[Plot] Grid and BG", enum."[Axis] Range X Scale", enum."[Axis] Range Y Scale", enum."[Axis] Axis and Label", enum."[Axis] Format String", enum."[Cursor] Appearance", enum."[Cursor] Index", enum."[Legend] Pair Strings", enum."[Legend] Checkbox", enum."[Legend] Tree Open", enum."[Legend] Color", enum."[Layout] Graph Type Change", enum."[Layout] Legend Visible Change", enum."[Layout] Update", enum."[Layout] Min Pane Size", enum."[Cursor] Cursor Info"] items=["None", "[Axis] Range X Scale", "[Axis] Range Y Scale", "[Layout] Graph Type Change", "[Plot] Tacho Point", "[Plot] Grid and BG", "[Cursor] Cursor Info", "[Legend] Pair Strings", "[Data] Plot Data", "[Legend] Checkbox", "[Layout] Update", "[Legend] Tree Open", "[Layout] Legend Visible Change", "[Plot] Data Point", "[Cursor] Appearance", "[Cursor] Index", "[Legend] Color", "[Axis] Axis and Label", "[Axis] Format String", "[Layout] Min Pane Size", "[Data] Index", "[Plot] Caption", "[Data] Legend Strings"]
            # "When an XCtrl is opened from file or copied from another XCtrl, initial state of the above\nproperty nodes of some facade elements should be restored, since we use these property\nnodes for '[Layout] Graph Type Change' and '[Layout] Legend Visible Change' update."
            n217 = Unbundle By Name(w472) -> ("Data Related State"=w473:T6)
            n218 = Dequeue Element(queue=w473) -> (queue out=w475:T6, element=w471:T13)  [unwired: 2 in, 2 out]
            n219 = Unbundle By Name(w471) -> ("Tree Visible?"=w480:bool, "Graph Type"=w479:T5)
            n220 = property on="Tree" class="Tree (strict)"("Visible"=w480) -> ()  [unwired: 2 in, 2 out]
            n221 = Bundle By Name(cluster=w471, "State Newer?"=TRUE ("Updated?")) -> (w476:T13)
            n222 = case shown="\"Probe X\", Default" w479 {
              tunnel: [TRUE FALSE w487] -> w478
              tunnel: [FALSE TRUE w487] -> w477
              frame "Probe X", Default {
              }
              frame "Probe Y" {
              }
              frame "Probe X and Y" {
                w487 = TRUE
              }
            }
            n223 = property on="Probe X" class="XYGraph (strict)"("Visible"=w478) -> ()  [unwired: 2 in, 2 out]
            n224 = property on="Probe Y" class="XYGraph (strict)"("Visible"=w477) -> ()  [unwired: 2 in, 2 out]
            n225 = Enqueue Element(queue=w475, element=w476) -> ()  [unwired: 2 in, 3 out]
          }
        }
      }
      event Direction Change {
        n226 = event-data() -> ()  [unwired: 1 in, 4 out]
      }
      event Exec State Change {
        n227 = event-data() -> ()  [unwired: 1 in, 4 out]
      }
      event Pane Size {
        w503 = T12[] [enum."[Layout] Update", enum."[Cursor] Cursor Info"] items=["None", "[Axis] Range X Scale", "[Axis] Range Y Scale", "[Layout] Graph Type Change", "[Plot] Tacho Point", "[Plot] Grid and BG", "[Cursor] Cursor Info", "[Legend] Pair Strings", "[Data] Plot Data", "[Legend] Checkbox", "[Layout] Update", "[Legend] Tree Open", "[Layout] Legend Visible Change", "[Plot] Data Point", "[Cursor] Appearance", "[Cursor] Index", "[Legend] Color", "[Axis] Axis and Label", "[Axis] Format String", "[Layout] Min Pane Size", "[Data] Index", "[Plot] Caption", "[Data] Legend Strings"] ("f")
        n228 = event-data() -> ("NewBnds.Right"=w508:i16, "NewBnds.Left"=w502:i16, "NewBnds.Bottom"=w509:i16, "NewBnds.Top"=w501:i16)  [unwired: 1 in]
        n229 = Unbundle By Name(w494) -> ("Data Related State"=w499:T6)
        n230 = Subtract(x=w508, y=w502) -> (x-y=w505:i16)
        n231 = Subtract(x=w509, y=w501) -> (x-y=w504:i16)
        n232 = Bundle By Name(cluster=T4 {"Width"=0, "Height"=0} ("Container Bounds"), "Width"=w505, "Height"=w504) -> (w495:T4)
        n233 = Dequeue Element(queue=w499) -> (queue out=w498:T6, element=w497:T13)  [unwired: 2 in, 2 out]
        n234 = Bundle By Name(cluster=w497, "Container Bounds"=w495) -> (w496:T13)
        n235 = Enqueue Element(queue=w498, element=w496) -> ()  [unwired: 2 in, 3 out]
      }
      event "Probe X", "Probe Y": Cursor Release {
        w519 = T12[] [enum."[Cursor] Index", enum."[Cursor] Cursor Info"] items=["None", "[Axis] Range X Scale", "[Axis] Range Y Scale", "[Layout] Graph Type Change", "[Plot] Tacho Point", "[Plot] Grid and BG", "[Cursor] Cursor Info", "[Legend] Pair Strings", "[Data] Plot Data", "[Legend] Checkbox", "[Layout] Update", "[Legend] Tree Open", "[Layout] Legend Visible Change", "[Plot] Data Point", "[Cursor] Appearance", "[Cursor] Index", "[Legend] Color", "[Axis] Axis and Label", "[Axis] Format String", "[Layout] Min Pane Size", "[Data] Index", "[Plot] Caption", "[Data] Legend Strings"] ("f")
        n236 = event-data() -> ("PointIdx"=w513:i32)  [unwired: 1 in]
        n237 = Unbundle By Name(w510) -> ("Data Related State"=w518:T6)
        n238 = Dequeue Element(queue=w518) -> (queue out=w517:T6, element=w515:T13)  [unwired: 2 in, 2 out]
        n239 = Unbundle By Name(w515) -> ("Index"=w516:cluster{"Pair Index":u32, "Order Index":u32}[])
        n240 = Index Array(array=w516) -> (element=w537:cluster{"Pair Index":u32, "Order Index":u32})  [unwired: 1 in]
        n241 = Unbundle By Name(w537) -> ("Pair Index"=w536:u32, "Order Index"=w535:u32)
        n242 = Index Array(array=w534, index (row)=w536, index (col)=w535) -> (element=w533:T15)
        n243 = Unbundle By Name(w533) -> ("reference"=w530:dbl[], "X"=w532:dbl[], "Y"=w531:dbl[])
        n244 = Bundle By Name(cluster=w527, "State Changed?"=TRUE, "Action Name"="Move") -> (w526:T2)
        n245 = Index Array(array=w530, index=w513) -> (element=w523:dbl)
        n246 = Index Array(array=w532, index=w513) -> (element=w522:dbl)
        n247 = Index Array(array=w531, index=w513) -> (element=w521:dbl)
        n248 = Bundle(w523, w522) -> (w512:cluster{dbl, dbl})  [unwired: 1 in]
        n249 = Bundle(w523, w521) -> (w511:cluster{dbl, dbl})  [unwired: 1 in]
        n250 = Bundle By Name(cluster=T10 {"PointIdx"=0, "Position"={"Probe X"=0.0, "Probe Y"=0.0, "Reference"=0.0}} ("event data"), "Position.Reference"=w523, "Position.Probe X"=w522, "Position.Probe Y"=w521, "PointIdx"=w513) -> (w520:T10)
        n251 = Bundle By Name(cluster=w515, "Cursor Index"=w513, "Cursor X Pos"=w512, "Cursor Y Pos"=w511) -> (w514:T13)
        n252 = Enqueue Element(queue=w517, element=w514) -> ()  [unwired: 2 in, 3 out]
        n253 = Unbundle By Name(w510) -> ("Cursor Release"=w525:refnum<user-event>)
        n254 = Generate User Event(user event=w525, event data cluster=w520) -> ()  [unwired: 2 in, 2 out]
      }
      event "Probe X", "Probe Y": Cursor Move {
        w547 = T12[] [enum."[Cursor] Index", enum."[Cursor] Cursor Info"] items=["None", "[Axis] Range X Scale", "[Axis] Range Y Scale", "[Layout] Graph Type Change", "[Plot] Tacho Point", "[Plot] Grid and BG", "[Cursor] Cursor Info", "[Legend] Pair Strings", "[Data] Plot Data", "[Legend] Checkbox", "[Layout] Update", "[Legend] Tree Open", "[Layout] Legend Visible Change", "[Plot] Data Point", "[Cursor] Appearance", "[Cursor] Index", "[Legend] Color", "[Axis] Axis and Label", "[Axis] Format String", "[Layout] Min Pane Size", "[Data] Index", "[Plot] Caption", "[Data] Legend Strings"] ("f")
        n255 = event-data() -> ("PointIdx"=w542:i32)  [unwired: 1 in]
        n256 = Unbundle By Name(w538) -> ("Data Related State"=w546:T6)
        n257 = Dequeue Element(queue=w546) -> (queue out=w545:T6, element=w544:T13)  [unwired: 2 in, 2 out]
        n258 = Unbundle By Name(w544) -> ("Index"=w539:cluster{"Pair Index":u32, "Order Index":u32}[])
        n259 = Index Array(array=w539) -> (element=w559:cluster{"Pair Index":u32, "Order Index":u32})  [unwired: 1 in]
        n260 = Unbundle By Name(w559) -> ("Pair Index"=w558:u32, "Order Index"=w557:u32)
        n261 = Index Array(array=w556, index (row)=w558, index (col)=w557) -> (element=w555:T15)
        n262 = Unbundle By Name(w555) -> ("reference"=w552:dbl[], "X"=w554:dbl[], "Y"=w553:dbl[])
        n263 = Index Array(array=w552, index=w542) -> (element=w549:dbl)
        n264 = Index Array(array=w554, index=w542) -> (element=w551:dbl)
        n265 = Index Array(array=w553, index=w542) -> (element=w550:dbl)
        n266 = Bundle(w549, w551) -> (w541:cluster{dbl, dbl})  [unwired: 1 in]
        n267 = Bundle(w549, w550) -> (w540:cluster{dbl, dbl})  [unwired: 1 in]
        n268 = Bundle By Name(cluster=w544, "Cursor Index"=w542, "Cursor X Pos"=w541, "Cursor Y Pos"=w540) -> (w543:T13)
        n269 = Enqueue Element(queue=w545, element=w543) -> ()  [unwired: 2 in, 3 out]
      }
      event "Probe X": Scale Range Change {
        n270 = event-data() -> ("NewRange.Maximum"=w575:dbl, "NewRange.Minimum"=w574:dbl, "Kind"=w569:enum16{"X-Scale", "Y-Scale", "Z-Scale"})  [unwired: 1 in]
        n271 = Unbundle By Name(w565) -> ("Data Related State"=w564:T6)
        n272 = Dequeue Element(queue=w564) -> (queue out=w560:T6, element=w563:T13)  [unwired: 2 in, 2 out]
        n273 = case shown="\"Y-Scale\"" w569 {
          tunnel: w565 -> [w590 w603]
          tunnel: [w589 w602] -> w576
          tunnel: [w588 w601] -> w567
          tunnel: w575 -> [w586 w598]
          tunnel: w574 -> [w585 w599]
          tunnel: [w584 w597] -> w566
          tunnel: w563 -> [w583 w595]
          tunnel: [w580 w594] -> w562
          tunnel: [w579 w596] -> w561
          tunnel: w560 -> [w579 w596]
          frame "Y-Scale" {
            w584 = T12[] [enum."[Axis] Range Y Scale"] items=["None", "[Axis] Range X Scale", "[Axis] Range Y Scale", "[Layout] Graph Type Change", "[Plot] Tacho Point", "[Plot] Grid and BG", "[Cursor] Cursor Info", "[Legend] Pair Strings", "[Data] Plot Data", "[Legend] Checkbox", "[Layout] Update", "[Legend] Tree Open", "[Layout] Legend Visible Change", "[Plot] Data Point", "[Cursor] Appearance", "[Cursor] Index", "[Legend] Color", "[Axis] Axis and Label", "[Axis] Format String", "[Layout] Min Pane Size", "[Data] Index", "[Plot] Caption", "[Data] Legend Strings"] ("f")
            w578 = FALSE ("X Scale.Autoscale")
            n274 = Max & Min(x=w586, y=w585) -> (max(x,y)=w582:dbl, min(x,y)=w581:dbl)
            n275 = Bundle By Name(cluster=w590, "Y Scale.Maximum.Probe X"=w582, "Y Scale.Minimum.Probe X"=w581, "Y Scale.Autoscale"=w578, "Y Scale.Autoscale Once"=w578) -> (w589:T3)
            n276 = Bundle By Name(cluster=w583, "Maximum.Probe X"=w582, "Minimum.Probe X"=w581) -> (w580:T13)
            n277 = Bundle By Name(cluster=T11 {"Minimum"=0.0, "Maximum"=0.0, "Kind"=enum."Y-Scale", "Graph Type"=enum."Probe X"} ("event data"), "Maximum"=w582, "Minimum"=w581) -> (w588:T11)
          }
          frame "X-Scale", Default {
            w597 = T12[] [enum."[Axis] Range X Scale"] items=["None", "[Axis] Range X Scale", "[Axis] Range Y Scale", "[Layout] Graph Type Change", "[Plot] Tacho Point", "[Plot] Grid and BG", "[Cursor] Cursor Info", "[Legend] Pair Strings", "[Data] Plot Data", "[Legend] Checkbox", "[Layout] Update", "[Legend] Tree Open", "[Layout] Legend Visible Change", "[Plot] Data Point", "[Cursor] Appearance", "[Cursor] Index", "[Legend] Color", "[Axis] Axis and Label", "[Axis] Format String", "[Layout] Min Pane Size", "[Data] Index", "[Plot] Caption", "[Data] Legend Strings"] ("f")
            w591 = FALSE ("X Scale.Autoscale")
            n278 = Max & Min(x=w598, y=w599) -> (max(x,y)=w593:dbl, min(x,y)=w592:dbl)
            n279 = Bundle By Name(cluster=w603, "X Scale.Maximum"=w593, "X Scale.Minimum"=w592, "X Scale.Autoscale"=w591, "X Scale.Autoscale Once"=w591) -> (w602:T3)
            n280 = Bundle By Name(cluster=w595, "Maximum"=w593, "Minimum"=w592) -> (w594:T13)
            n281 = Bundle By Name(cluster=T11 {"Minimum"=0.0, "Maximum"=0.0, "Kind"=enum."X-Scale", "Graph Type"=enum."Probe X and Y"} ("event data"), "Maximum"=w593, "Minimum"=w592) -> (w601:T11)
          }
        }
        n282 = Bundle By Name(cluster=w571, "Action Name"="Range Changed", "State Changed?"=TRUE) -> (w570:T2)
        n283 = Unbundle By Name(w576) -> ("Scale Range Change"=w568:refnum<user-event>)
        n284 = Enqueue Element(queue=w561, element=w562) -> ()  [unwired: 2 in, 3 out]
        n285 = Generate User Event(user event=w568, event data cluster=w567) -> ()  [unwired: 2 in, 2 out]
      }
      event "Probe Y": Scale Range Change {
        n286 = event-data() -> ("NewRange.Maximum"=w617:dbl, "NewRange.Minimum"=w616:dbl, "Kind"=w611:enum16{"X-Scale", "Y-Scale", "Z-Scale"})  [unwired: 1 in]
        n287 = Unbundle By Name(w609) -> ("Data Related State"=w608:T6)
        n288 = Dequeue Element(queue=w608) -> (queue out=w607:T6, element=w606:T13)  [unwired: 2 in, 2 out]
        n289 = case shown="\"X-Scale\", Default" w611 {
          tunnel: w609 -> [w634 w647]
          tunnel: [w633 w646] -> w620
          tunnel: [w632 w645] -> w618
          tunnel: w617 -> [w630 w643]
          tunnel: w616 -> [w629 w642]
          tunnel: [w628 w641] -> w610
          tunnel: w607 -> [w627 w640]
          tunnel: w606 -> [w626 w639]
          tunnel: [w627 w640] -> w605
          tunnel: [w625 w638] -> w604
          frame "Y-Scale" {
            w628 = T12[] [enum."[Axis] Range Y Scale"] items=["None", "[Axis] Range X Scale", "[Axis] Range Y Scale", "[Layout] Graph Type Change", "[Plot] Tacho Point", "[Plot] Grid and BG", "[Cursor] Cursor Info", "[Legend] Pair Strings", "[Data] Plot Data", "[Legend] Checkbox", "[Layout] Update", "[Legend] Tree Open", "[Layout] Legend Visible Change", "[Plot] Data Point", "[Cursor] Appearance", "[Cursor] Index", "[Legend] Color", "[Axis] Axis and Label", "[Axis] Format String", "[Layout] Min Pane Size", "[Data] Index", "[Plot] Caption", "[Data] Legend Strings"] ("f")
            w622 = FALSE ("X Scale.Autoscale")
            n290 = Max & Min(x=w630, y=w629) -> (max(x,y)=w624:dbl, min(x,y)=w623:dbl)
            n291 = Bundle By Name(cluster=w634, "Y Scale.Maximum.Probe Y"=w624, "Y Scale.Minimum.Probe Y"=w623, "Y Scale.Autoscale"=w622, "Y Scale.Autoscale Once"=w622) -> (w633:T3)
            n292 = Bundle By Name(cluster=w626, "Maximum.Probe Y"=w624, "Minimum.Probe Y"=w623) -> (w625:T13)
            n293 = Bundle By Name(cluster=T11 {"Minimum"=0.0, "Maximum"=0.0, "Kind"=enum."Y-Scale", "Graph Type"=enum."Probe Y"} ("event data"), "Maximum"=w624, "Minimum"=w623) -> (w632:T11)
          }
          frame "X-Scale", Default {
            w641 = T12[] [enum."[Axis] Range X Scale"] items=["None", "[Axis] Range X Scale", "[Axis] Range Y Scale", "[Layout] Graph Type Change", "[Plot] Tacho Point", "[Plot] Grid and BG", "[Cursor] Cursor Info", "[Legend] Pair Strings", "[Data] Plot Data", "[Legend] Checkbox", "[Layout] Update", "[Legend] Tree Open", "[Layout] Legend Visible Change", "[Plot] Data Point", "[Cursor] Appearance", "[Cursor] Index", "[Legend] Color", "[Axis] Axis and Label", "[Axis] Format String", "[Layout] Min Pane Size", "[Data] Index", "[Plot] Caption", "[Data] Legend Strings"] ("f")
            w635 = FALSE ("X Scale.Autoscale")
            n294 = Max & Min(x=w643, y=w642) -> (max(x,y)=w637:dbl, min(x,y)=w636:dbl)
            n295 = Bundle By Name(cluster=w647, "X Scale.Maximum"=w637, "X Scale.Minimum"=w636, "X Scale.Autoscale"=w635, "X Scale.Autoscale Once"=w635) -> (w646:T3)
            n296 = Bundle By Name(cluster=T11 {"Minimum"=0.0, "Maximum"=0.0, "Kind"=enum."X-Scale", "Graph Type"=enum."Probe X and Y"} ("event data"), "Maximum"=w637, "Minimum"=w636) -> (w645:T11)
            n297 = Bundle By Name(cluster=w639, "Maximum"=w637, "Minimum"=w636) -> (w638:T13)
          }
        }
        n298 = Bundle By Name(cluster=w613, "Action Name"="Range Changed", "State Changed?"=TRUE) -> (w612:T2)
        n299 = Unbundle By Name(w620) -> ("Scale Range Change"=w619:refnum<user-event>)
        n300 = Enqueue Element(queue=w605, element=w604) -> ()  [unwired: 2 in, 3 out]
        n301 = Generate User Event(user event=w619, event data cluster=w618) -> ()  [unwired: 2 in, 2 out]
      }
      event Shortcut Menu Activation? {
        n302 = event-data() -> ("Coords"=w650:T1)  [unwired: 1 in]
        n303 = control-ref of="Probe X"() -> (w649:refnum<vi>)
        n304 = control-ref of="Probe Y"() -> (w648:refnum<vi>)
        n305 = call <vilib>:"svx_Timebase Pane SCMenuDiscard.vi"("Coords"=w650, "Probe Y"=w648, "Probe X"=w649) -> ("Boolean"=w651:bool)  [unwired: 8 in]
        n306 = local write "Coords"(w650) -> ()
        n307 = event-data("Discard?"=w651) -> ()  [unwired: 1 in, 1 out]
      }
      event "Probe X", "Probe Y": Shortcut Menu Activation? {
        n308 = event-data() -> ("MenuRef"=w661:refnum<k9>, "Coords"=→"Coords":T1)  [unwired: 1 in]
        n309 = Unbundle By Name(w662) -> ("Refnum"=w656:refnum<vi>, "Run Mode?"=w657:bool)
        n310 = call <vilib>:"svx_Timebase SC Menu.vi"("Run Mode?"=w657, "State"=w660, "Refnum"=w656, "MenuRef"=w661) -> ()  [unwired: 8 in]
        n311 = event-data() -> ()  [unwired: 2 in, 1 out]
      }
      event "Probe X", "Probe Y": Shortcut Menu Selection? (App) {
        n312 = event-data() -> ("ItemTag"=w671:string)  [unwired: 1 in]
        n313 = case shown="Default" w671 {
          tunnel: w667 -> [w676 w686]
          tunnel: [w672 w682] -> w663
          tunnel: [w676 w685] -> w666
          tunnel: w670 -> [w674 _]
          tunnel: [FALSE ("Discard?") TRUE ("Discard?")] -> w668
          tunnel: [w674 T8 [] ("timebase plot")] -> w669
          tunnel: w665 -> [w673 w679]
          tunnel: [w673 w678] -> w664
          frame Default {
            w672 = T12[] [] items=["None", "[Axis] Range X Scale", "[Axis] Range Y Scale", "[Layout] Graph Type Change", "[Plot] Tacho Point", "[Plot] Grid and BG", "[Cursor] Cursor Info", "[Legend] Pair Strings", "[Data] Plot Data", "[Legend] Checkbox", "[Layout] Update", "[Legend] Tree Open", "[Layout] Legend Visible Change", "[Plot] Data Point", "[Cursor] Appearance", "[Cursor] Index", "[Legend] Color", "[Axis] Axis and Label", "[Axis] Format String", "[Layout] Min Pane Size", "[Data] Index", "[Plot] Caption", "[Data] Legend Strings"]
          }
          frame "APP_SC_CLEAR_GRAPH" {
            w680 = string[] [] ("Strings[].row strings []")
            w682 = T12[] [enum."[Data] Plot Data", enum."[Data] Legend Strings", enum."[Cursor] Cursor Info", enum."[Legend] Pair Strings", enum."[Legend] Checkbox", enum."[Legend] Tree Open"] items=["None", "[Axis] Range X Scale", "[Axis] Range Y Scale", "[Layout] Graph Type Change", "[Plot] Tacho Point", "[Plot] Grid and BG", "[Cursor] Cursor Info", "[Legend] Pair Strings", "[Data] Plot Data", "[Legend] Checkbox", "[Layout] Update", "[Legend] Tree Open", "[Layout] Legend Visible Change", "[Plot] Data Point", "[Cursor] Appearance", "[Cursor] Index", "[Legend] Color", "[Axis] Axis and Label", "[Axis] Format String", "[Layout] Min Pane Size", "[Data] Index", "[Plot] Caption", "[Data] Legend Strings"]
            w681 = TRUE ("State Changed?")
            n314 = Bundle By Name(cluster=w686, "Action Name"="Clear Graph", "Data Changed?"=w681, "State Changed?"=w681) -> (w685:T2)
            n315 = Bundle By Name(cluster=w679, "Strings[].Row Strings []"=w680, "Strings[].Column Strings []"=w680) -> (w678:T3)
          }
        }
        n316 = event-data("Discard?"=w668) -> ()  [unwired: 1 in, 1 out]
      }
      event "Probe X", "Probe Y": Shortcut Menu Selection (User) {
        n317 = event-data() -> ("CtlRef"=w688:refnum<vi>, "ItemTag"=w696:string)  [unwired: 1 in]
        n318 = Unbundle By Name(w690) -> ("Refnum"=w689:refnum<vi>)
        n319 = case shown="\"USER_SC_SELECTOR\"" w696 {
          tunnel: w689 -> [_ w704 w710 _ _ _ _ _ _ _ w791 _ _ _ _ _]
          tunnel: w691 -> [w698 w700 w706 w718 w727 w736 w740 w749 w764 w772 w793 w803 w815 w827 w837 w846]
          tunnel: [_ _ _ w711 w720 w729 w743 w752 w762 w769 _ w800 w812 w824 w838 w847] -> w687
          tunnel: w695 -> [w697 w699 w705 w713 w722 w731 w746 w755 w768 w777 w782 w796 w807 w819 w833 w842]
          tunnel: [w697 w699 w705 w719 w728 w737 w745 w754 w767 w776 w779 w801 w813 w825 w831 w840] -> w694
          tunnel: [w698 w700 w706 w717 w726 w735 w739 w748 w763 w771 w792 w802 w814 w826 w836 w845] -> w692
          tunnel: w693 -> [_ _ _ _ _ _ _ _ _ _ w778 _ _ _ _ _]
          tunnel: w688 -> [_ _ _ _ _ _ _ _ _ _ _ _ _ _ _ _]
          frame "False", Default {
          }
          frame "USER_SC_LABEL" {
            n320 = property class="Ctl"(reference=w704) -> (reference out=w701:refnum<vi>, "Label.Visible"=w703:bool)  [unwired: 1 in, 1 out]
            n321 = Not(x=w703) -> (.not. x?=w702:bool)
            n322 = property class="Ctl"(reference=w701, "Label.Visible"=w702) -> ()  [unwired: 1 in, 2 out]
          }
          frame "USER_SC_CAPTION" {
            n323 = property class="Ctl"(reference=w710) -> (reference out=w707:refnum<vi>, "Caption.Visible"=w709:bool)  [unwired: 1 in, 1 out]
            n324 = Not(x=w709) -> (.not. x?=w708:bool)
            n325 = property class="Ctl"(reference=w707, "Caption.Visible"=w708) -> ()  [unwired: 1 in, 2 out]
          }
          frame "USER_SC_X_SCALE_PROBEX" {
            w711 = T12[] [enum."[Axis] Axis and Label"] items=["None", "[Axis] Range X Scale", "[Axis] Range Y Scale", "[Layout] Graph Type Change", "[Plot] Tacho Point", "[Plot] Grid and BG", "[Cursor] Cursor Info", "[Legend] Pair Strings", "[Data] Plot Data", "[Legend] Checkbox", "[Layout] Update", "[Legend] Tree Open", "[Layout] Legend Visible Change", "[Plot] Data Point", "[Cursor] Appearance", "[Cursor] Index", "[Legend] Color", "[Axis] Axis and Label", "[Axis] Format String", "[Layout] Min Pane Size", "[Data] Index", "[Plot] Caption", "[Data] Legend Strings"] ("f")
            n326 = Unbundle By Name(w713) -> ("X Scale.Show Scale.Probe X"=w712:bool)
            n327 = Bundle By Name(cluster=w718, "Action Name"="Show/Hide", "State Changed?"=TRUE) -> (w717:T2)
            n328 = Not(x=w712) -> (.not. x?=w714:bool)
            n329 = Bundle By Name(cluster=w713, "X Scale.Show Scale.Probe X"=w714) -> (w719:T3)
          }
          frame "USER_SC_X_SCALE_PROBEY" {
            w720 = T12[] [enum."[Axis] Axis and Label"] items=["None", "[Axis] Range X Scale", "[Axis] Range Y Scale", "[Layout] Graph Type Change", "[Plot] Tacho Point", "[Plot] Grid and BG", "[Cursor] Cursor Info", "[Legend] Pair Strings", "[Data] Plot Data", "[Legend] Checkbox", "[Layout] Update", "[Legend] Tree Open", "[Layout] Legend Visible Change", "[Plot] Data Point", "[Cursor] Appearance", "[Cursor] Index", "[Legend] Color", "[Axis] Axis and Label", "[Axis] Format String", "[Layout] Min Pane Size", "[Data] Index", "[Plot] Caption", "[Data] Legend Strings"] ("f")
            n330 = Unbundle By Name(w722) -> ("X Scale.Show Scale.Probe Y"=w721:bool)
            n331 = Bundle By Name(cluster=w727, "Action Name"="Show/Hide", "State Changed?"=TRUE) -> (w726:T2)
            n332 = Not(x=w721) -> (.not. x?=w723:bool)
            n333 = Bundle By Name(cluster=w722, "X Scale.Show Scale.Probe Y"=w723) -> (w728:T3)
          }
          frame "USER_SC_Y_SCALE" {
            w729 = T12[] [enum."[Axis] Axis and Label"] items=["None", "[Axis] Range X Scale", "[Axis] Range Y Scale", "[Layout] Graph Type Change", "[Plot] Tacho Point", "[Plot] Grid and BG", "[Cursor] Cursor Info", "[Legend] Pair Strings", "[Data] Plot Data", "[Legend] Checkbox", "[Layout] Update", "[Legend] Tree Open", "[Layout] Legend Visible Change", "[Plot] Data Point", "[Cursor] Appearance", "[Cursor] Index", "[Legend] Color", "[Axis] Axis and Label", "[Axis] Format String", "[Layout] Min Pane Size", "[Data] Index", "[Plot] Caption", "[Data] Legend Strings"] ("f")
            n334 = Unbundle By Name(w731) -> ("Y Scale.Scale Visible"=w730:bool)
            n335 = Bundle By Name(cluster=w736, "Action Name"="Show/Hide", "State Changed?"=TRUE) -> (w735:T2)
            n336 = Not(x=w730) -> (.not. x?=w732:bool)
            n337 = Bundle By Name(cluster=w731, "Y Scale.Scale Visible"=w732) -> (w737:T3)
          }
          frame "USER_SC_CURSOR" {
            w743 = T12[] [enum."[Cursor] Cursor Info"] items=["None", "[Axis] Range X Scale", "[Axis] Range Y Scale", "[Layout] Graph Type Change", "[Plot] Tacho Point", "[Plot] Grid and BG", "[Cursor] Cursor Info", "[Legend] Pair Strings", "[Data] Plot Data", "[Legend] Checkbox", "[Layout] Update", "[Legend] Tree Open", "[Layout] Legend Visible Change", "[Plot] Data Point", "[Cursor] Appearance", "[Cursor] Index", "[Legend] Color", "[Axis] Axis and Label", "[Axis] Format String", "[Layout] Min Pane Size", "[Data] Index", "[Plot] Caption", "[Data] Legend Strings"] ("f")
            n338 = Unbundle By Name(w746) -> ("Cursor.Cursor Visible"=w744:bool)
            n339 = Bundle By Name(cluster=w740, "Action Name"="Show Cursor", "State Changed?"=TRUE) -> (w739:T2)
            n340 = Not(x=w744) -> (.not. x?=w738:bool)
            n341 = Bundle By Name(cluster=w746, "Cursor.Cursor Visible"=w738) -> (w745:T3)
          }
          frame "USER_SC_CURSOR_INFO" {
            w752 = T12[] [enum."[Cursor] Cursor Info"] items=["None", "[Axis] Range X Scale", "[Axis] Range Y Scale", "[Layout] Graph Type Change", "[Plot] Tacho Point", "[Plot] Grid and BG", "[Cursor] Cursor Info", "[Legend] Pair Strings", "[Data] Plot Data", "[Legend] Checkbox", "[Layout] Update", "[Legend] Tree Open", "[Layout] Legend Visible Change", "[Plot] Data Point", "[Cursor] Appearance", "[Cursor] Index", "[Legend] Color", "[Axis] Axis and Label", "[Axis] Format String", "[Layout] Min Pane Size", "[Data] Index", "[Plot] Caption", "[Data] Legend Strings"] ("f")
            n342 = Unbundle By Name(w755) -> ("Cursor.Cursor Name Visible"=w753:bool)
            n343 = Not(x=w753) -> (.not. x?=w747:bool)
            n344 = Bundle By Name(cluster=w749, "Action Name"="Show Cursor Info", "State Changed?"=TRUE) -> (w748:T2)
            n345 = Bundle By Name(cluster=w755, "Cursor.Cursor Name Visible"=w747) -> (w754:T3)
          }
          frame "USER_SC_SELECTOR" {
            w762 = T12[] [enum."[Layout] Legend Visible Change", enum."[Layout] Update", enum."[Layout] Min Pane Size"] items=["None", "[Axis] Range X Scale", "[Axis] Range Y Scale", "[Layout] Graph Type Change", "[Plot] Tacho Point", "[Plot] Grid and BG", "[Cursor] Cursor Info", "[Legend] Pair Strings", "[Data] Plot Data", "[Legend] Checkbox", "[Layout] Update", "[Legend] Tree Open", "[Layout] Legend Visible Change", "[Plot] Data Point", "[Cursor] Appearance", "[Cursor] Index", "[Legend] Color", "[Axis] Axis and Label", "[Axis] Format String", "[Layout] Min Pane Size", "[Data] Index", "[Plot] Caption", "[Data] Legend Strings"] ("f")
            n346 = Unbundle By Name(w768) -> ("Legend Visible"=w761:bool, "Data Related State"=w757:T6)
            n347 = Dequeue Element(queue=w757) -> (queue out=w759:T6, element=w760:T13)  [unwired: 2 in, 2 out]
            n348 = Bundle By Name(cluster=w764, "Action Name"="Show Selector", "State Changed?"=TRUE) -> (w763:T2)
            n349 = Not(x=w761) -> (.not. x?=w756:bool)
            n350 = Bundle By Name(cluster=w760, "Tree Visible?"=w756) -> (w758:T13)
            n351 = Bundle By Name(cluster=w768, "Legend Visible"=w756) -> (w767:T3)
            n352 = Enqueue Element(queue=w759, element=w758) -> ()  [unwired: 2 in, 3 out]
          }
          frame "USER_SC_LOCK" {
            w769 = T12[] [enum."[Cursor] Cursor Info"] items=["None", "[Axis] Range X Scale", "[Axis] Range Y Scale", "[Layout] Graph Type Change", "[Plot] Tacho Point", "[Plot] Grid and BG", "[Cursor] Cursor Info", "[Legend] Pair Strings", "[Data] Plot Data", "[Legend] Checkbox", "[Layout] Update", "[Legend] Tree Open", "[Layout] Legend Visible Change", "[Plot] Data Point", "[Cursor] Appearance", "[Cursor] Index", "[Legend] Color", "[Axis] Axis and Label", "[Axis] Format String", "[Layout] Min Pane Size", "[Data] Index", "[Plot] Caption", "[Data] Legend Strings"] ("f")
            n353 = Unbundle By Name(w777) -> ("Cursor.Cursor Lock"=w775:bool)
            n354 = Bundle By Name(cluster=w772, "Action Name"="Lock Cursor", "State Changed?"=TRUE) -> (w771:T2)
            n355 = Not(x=w775) -> (.not. x?=w770:bool)
            n356 = Bundle By Name(cluster=w777, "Cursor.Cursor Lock"=w770) -> (w776:T3)
          }
          frame "USER_SC_PROPERTIES" {
            n357 = control-ref of="Probe X"() -> (w790:refnum<vi>)
            n358 = control-ref of="Probe Y"() -> (w789:refnum<vi>)
            n359 = control-ref of="Tree"() -> (w788:refnum<vi>)
            n360 = control-ref of="Split"() -> (w787:refnum<vi>)
            n361 = control-ref of="cursor X info"() -> (w786:refnum<vi>)
            n362 = control-ref of="cursor Y info"() -> (w785:refnum<vi>)
            n363 = control-ref of="This VI"() -> (w783:refnum<vi>)
            n364 = Bundle("Probe X"=w790, "Probe Y"=w789, "Tree"=w788, "Split"=w787, "cursor X info"=w786, "cursor Y info"=w785) -> (w784:T16)  [unwired: 1 in]
            n365 = call <vilib>:"svx_Timebase Queue To State.vi"("Display State In"=w782) -> ("Display State Out"=w781:T3)  [unwired: 10 in]
            n366 = call <vilib>:"svx_Timebase Property Dialog.vi"("Container"=w791, "Data"=w778, "State in"=w781, "Ref Ins"=w784, "Facade VI"=w783, "Action in"=w793) -> ("State out"=w780:T3, "Action out"=w792:T2)  [unwired: 8 in]
            n367 = call <vilib>:"svx_Timebase State To Queue.vi"("Display State In"=w780) -> ("Display State Out"=w779:T3)  [unwired: 10 in]
          }
          frame "USER_SC_SHOW_X" {
            w800 = T12[] [enum."[Layout] Graph Type Change", enum."[Layout] Update", enum."[Layout] Min Pane Size", enum."[Cursor] Cursor Info"] items=["None", "[Axis] Range X Scale", "[Axis] Range Y Scale", "[Layout] Graph Type Change", "[Plot] Tacho Point", "[Plot] Grid and BG", "[Cursor] Cursor Info", "[Legend] Pair Strings", "[Data] Plot Data", "[Legend] Checkbox", "[Layout] Update", "[Legend] Tree Open", "[Layout] Legend Visible Change", "[Plot] Data Point", "[Cursor] Appearance", "[Cursor] Index", "[Legend] Color", "[Axis] Axis and Label", "[Axis] Format String", "[Layout] Min Pane Size", "[Data] Index", "[Plot] Caption", "[Data] Legend Strings"] ("f")
            w794 = svx_Timebase_Graph_Types."Probe X" ("Graph Type")
            n368 = Unbundle By Name(w796) -> ("Data Related State"=w795:T6)
            n369 = Dequeue Element(queue=w795) -> (queue out=w798:T6, element=w799:T13)  [unwired: 2 in, 2 out]
            n370 = Bundle By Name(cluster=w803, "Action Name"="Graph Type Change", "State Changed?"=TRUE) -> (w802:T2)
            n371 = Bundle By Name(cluster=w799, "Graph Type"=w794) -> (w797:T13)
            n372 = Bundle By Name(cluster=w796, "Graph Type"=w794) -> (w801:T3)
            n373 = Enqueue Element(queue=w798, element=w797) -> ()  [unwired: 2 in, 3 out]
          }
          frame "USER_SC_SHOW_Y" {
            w812 = T12[] [enum."[Layout] Graph Type Change", enum."[Layout] Update", enum."[Layout] Min Pane Size", enum."[Cursor] Cursor Info"] items=["None", "[Axis] Range X Scale", "[Axis] Range Y Scale", "[Layout] Graph Type Change", "[Plot] Tacho Point", "[Plot] Grid and BG", "[Cursor] Cursor Info", "[Legend] Pair Strings", "[Data] Plot Data", "[Legend] Checkbox", "[Layout] Update", "[Legend] Tree Open", "[Layout] Legend Visible Change", "[Plot] Data Point", "[Cursor] Appearance", "[Cursor] Index", "[Legend] Color", "[Axis] Axis and Label", "[Axis] Format String", "[Layout] Min Pane Size", "[Data] Index", "[Plot] Caption", "[Data] Legend Strings"] ("f")
            w806 = svx_Timebase_Graph_Types."Probe Y" ("Graph Type")
            n374 = Unbundle By Name(w807) -> ("Data Related State"=w808:T6)
            n375 = Bundle By Name(cluster=w815, "Action Name"="Graph Type Change", "State Changed?"=TRUE) -> (w814:T2)
            n376 = Dequeue Element(queue=w808) -> (queue out=w810:T6, element=w811:T13)  [unwired: 2 in, 2 out]
            n377 = Bundle By Name(cluster=w811, "Graph Type"=w806) -> (w809:T13)
            n378 = Bundle By Name(cluster=w807, "Graph Type"=w806) -> (w813:T3)
            n379 = Enqueue Element(queue=w810, element=w809) -> ()  [unwired: 2 in, 3 out]
          }
          frame "USER_SC_SHOW_XY" {
            w824 = T12[] [enum."[Layout] Graph Type Change", enum."[Layout] Update", enum."[Layout] Min Pane Size", enum."[Cursor] Cursor Info"] items=["None", "[Axis] Range X Scale", "[Axis] Range Y Scale", "[Layout] Graph Type Change", "[Plot] Tacho Point", "[Plot] Grid and BG", "[Cursor] Cursor Info", "[Legend] Pair Strings", "[Data] Plot Data", "[Legend] Checkbox", "[Layout] Update", "[Legend] Tree Open", "[Layout] Legend Visible Change", "[Plot] Data Point", "[Cursor] Appearance", "[Cursor] Index", "[Legend] Color", "[Axis] Axis and Label", "[Axis] Format String", "[Layout] Min Pane Size", "[Data] Index", "[Plot] Caption", "[Data] Legend Strings"] ("f")
            w818 = svx_Timebase_Graph_Types."Probe X and Y" ("Graph Type")
            n380 = Unbundle By Name(w819) -> ("Data Related State"=w820:T6)
            n381 = Bundle By Name(cluster=w827, "Action Name"="Graph Type Change", "State Changed?"=TRUE) -> (w826:T2)
            n382 = Dequeue Element(queue=w820) -> (queue out=w822:T6, element=w823:T13)  [unwired: 2 in, 2 out]
            n383 = Bundle By Name(cluster=w823, "Graph Type"=w818) -> (w821:T13)
            n384 = Bundle By Name(cluster=w819, "Graph Type"=w818) -> (w825:T3)
            n385 = Enqueue Element(queue=w822, element=w821) -> ()  [unwired: 2 in, 3 out]
          }
          frame "USER_SC_AUTOSCALE_X" {
            w838 = T12[] [enum."[Axis] Range X Scale"] items=["None", "[Axis] Range X Scale", "[Axis] Range Y Scale", "[Layout] Graph Type Change", "[Plot] Tacho Point", "[Plot] Grid and BG", "[Cursor] Cursor Info", "[Legend] Pair Strings", "[Data] Plot Data", "[Legend] Checkbox", "[Layout] Update", "[Legend] Tree Open", "[Layout] Legend Visible Change", "[Plot] Data Point", "[Cursor] Appearance", "[Cursor] Index", "[Legend] Color", "[Axis] Axis and Label", "[Axis] Format String", "[Layout] Min Pane Size", "[Data] Index", "[Plot] Caption", "[Data] Legend Strings"] ("f")
            n386 = Unbundle By Name(w833) -> ("X Scale.Autoscale"=w834:bool)
            n387 = Bundle By Name(cluster=w837, "Action Name"="Graph Scale Option", "State Changed?"=TRUE) -> (w836:T2)
            n388 = Not(x=w834) -> (.not. x?=w832:bool)
            n389 = Bundle By Name(cluster=w833, "X Scale.Autoscale"=w832) -> (w831:T3)
          }
          frame "USER_SC_AUTOSCALE_Y" {
            w847 = T12[] [enum."[Axis] Range Y Scale"] items=["None", "[Axis] Range X Scale", "[Axis] Range Y Scale", "[Layout] Graph Type Change", "[Plot] Tacho Point", "[Plot] Grid and BG", "[Cursor] Cursor Info", "[Legend] Pair Strings", "[Data] Plot Data", "[Legend] Checkbox", "[Layout] Update", "[Legend] Tree Open", "[Layout] Legend Visible Change", "[Plot] Data Point", "[Cursor] Appearance", "[Cursor] Index", "[Legend] Color", "[Axis] Axis and Label", "[Axis] Format String", "[Layout] Min Pane Size", "[Data] Index", "[Plot] Caption", "[Data] Legend Strings"] ("f")
            n390 = Unbundle By Name(w842) -> ("Y Scale.Autoscale"=w843:bool)
            n391 = Bundle By Name(cluster=w846, "Action Name"="Graph Scale Option", "State Changed?"=TRUE) -> (w845:T2)
            n392 = Not(x=w843) -> (.not. x?=w841:bool)
            n393 = Bundle By Name(cluster=w842, "Y Scale.Autoscale"=w841) -> (w840:T3)
          }
        }
      }
      event "Split", "Tree": Shortcut Menu Activation? {
        n394 = event-data() -> ("Coords"=w848:T1)  [unwired: 1 in, 6 out]
        n395 = local write "Coords"(w848) -> ()
        n396 = event-data("Discard?"=TRUE) -> ()  [unwired: 1 in, 1 out]
      }
      event "Probe X", "Probe Y": Mouse Down {
        n397 = event-data() -> ("CtlRef"=w861:refnum<vi>, "Button"=w854:u16)  [unwired: 1 in]
        n398 = Equal?(x=w854, y=u16 1 ("x")) -> (x = y?=w862:bool)
        n399 = case shown="True" w862 {
          tunnel: w860 -> [w864 w884]
          tunnel: [w864 w883] -> w858
          tunnel: [w863 w881] -> w856
          tunnel: w859 -> [w863 w882]
          tunnel: w861 -> [_ w880]
          tunnel: [_ w879] -> w853
          frame False {
          }
          frame True {
            n400 = Unbundle By Name(w884) -> ("Background color"=w891:u32, "X Scale.Grid Style"=w874:u16, "X Scale.Major Color"=w873:u32, "X Scale.Minor Color"=w872:u32, "Y Scale.Grid Style"=w869:u16, "Y Scale.Major Color"=w868:u32, "Y Scale.Minor Color"=w867:u32)
            n401 = property on="Property Node" class="XYGraph (strict)"(reference=w880) -> ("BG Color"=w890:u32, "XScale.MajGrdColor"=w889:u32, "XScale.MnrGrdColor"=w888:u32, "YScale.MajGrdColor"=w887:u32, "YScale.MnrGrdColor"=w886:u32)  [unwired: 1 in, 2 out]
            n402 = case shown="0, Default" w869 {
              tunnel: w868 -> [_ w893 w896]
              tunnel: w867 -> [_ _ w895]
              tunnel: [w892 w893 w896] -> w866
              tunnel: [w892 u32 16777216 w895] -> w865
              frame 0, Default {
                w892 = u32 16777216
              }
              frame 1 {
              }
              frame 2 {
              }
            }
            n403 = case shown="0, Default" w874 {
              tunnel: w873 -> [_ w898 w901]
              tunnel: w872 -> [_ _ w900]
              tunnel: [w897 w898 w901] -> w871
              tunnel: [w897 u32 16777216 w900] -> w870
              frame 0, Default {
                w897 = u32 16777216
              }
              frame 1 {
              }
              frame 2 {
              }
            }
            n404 = Bundle("Background color"=w891, "Major Color"=w871, "Minor Color"=w870, "Major Color"=w866, "Minor Color"=w865) -> (w878:T17)  [unwired: 1 in]
            n405 = Bundle("BG Color"=w890, "XScale.MajGrdColor"=w889, "XScale.MnrGrdColor"=w888, "YScale.MajGrdColor"=w887, "YScale.MnrGrdColor"=w886) -> (w885:T18)  [unwired: 1 in]
            n406 = Not Equal?(x=w878, y=w885) -> (x != y?=w875:cluster{bool, bool, bool, bool, bool})
            n407 = Cluster To Array(cluster=w875) -> (array=w876:bool[])
            n408 = Or Array Elements(Boolean array=w876) -> (logical OR=w877:bool)
            n409 = case shown="True" w877 {
              tunnel: w885 -> [_ w919]
              tunnel: w884 -> [w903 w921]
              tunnel: [w903 w920] -> w883
              tunnel: w882 -> [w902 w918]
              tunnel: [w902 w917] -> w881
              tunnel: [_ w909] -> w879
              tunnel: w875 -> [_ w908]
              frame False {
              }
              frame True {
                w909 = T12[] [enum."[Plot] Grid and BG"] items=["None", "[Axis] Range X Scale", "[Axis] Range Y Scale", "[Layout] Graph Type Change", "[Plot] Tacho Point", "[Plot] Grid and BG", "[Cursor] Cursor Info", "[Legend] Pair Strings", "[Data] Plot Data", "[Legend] Checkbox", "[Layout] Update", "[Legend] Tree Open", "[Layout] Legend Visible Change", "[Plot] Data Point", "[Cursor] Appearance", "[Cursor] Index", "[Legend] Color", "[Axis] Axis and Label", "[Axis] Format String", "[Layout] Min Pane Size", "[Data] Index", "[Plot] Caption", "[Data] Legend Strings"] ("f")
                n410 = Unbundle(w908) -> (w907:bool, w906:bool, w905:bool)  [unwired: 2 out]
                n411 = Unbundle(w919) -> ("BG Color"=w914:u32, "XScale.MajGrdColor"=w913:u32, "XScale.MnrGrdColor"=w912:u32, "YScale.MajGrdColor"=w911:u32, "YScale.MnrGrdColor"=w910:u32)
                n412 = Or(x=w906, y=w905) -> (x .or. y?=w904:bool)
                n413 = case shown="False" w907 {
                  tunnel: w921 -> [w924 w931]
                  tunnel: [w923 w930] -> w920
                  tunnel: w914 -> [w922 _]
                  tunnel: w913 -> [_ w925]
                  tunnel: w912 -> [_ w926]
                  tunnel: w911 -> [_ w928]
                  tunnel: w910 -> [_ w927]
                  tunnel: w904 -> [_ w929]
                  frame True {
                    n414 = Bundle By Name(cluster=w924, "Background color"=w922) -> (w923:T3)
                  }
                  frame False {
                    n415 = case shown="False" w929 {
                      tunnel: w931 -> [w936 w941]
                      tunnel: [w935 w940] -> w930
                      tunnel: w928 -> [_ w938]
                      tunnel: w927 -> [_ w937]
                      tunnel: w926 -> [w933 _]
                      tunnel: w925 -> [w932 _]
                      frame True {
                        n416 = Bundle By Name(cluster=w936, "X Scale.Major Color"=w932, "X Scale.Minor Color"=w933, "X Scale.Grid Style"=u16 2) -> (w935:T3)
                      }
                      frame False {
                        n417 = Bundle By Name(cluster=w941, "Y Scale.Major Color"=w938, "Y Scale.Minor Color"=w937, "Y Scale.Grid Style"=u16 2 ("X Scale.Grid Style")) -> (w940:T3)
                      }
                    }
                  }
                }
                n418 = Bundle By Name(cluster=w918, "State Changed?"=TRUE, "Action Name"="Color Changed") -> (w917:T2)
              }
            }
          }
        }
      }
      event "Tree": event #0x1e; "Tree": Item Close {
        w942 = T12[] [enum."[Legend] Tree Open"] items=["None", "[Axis] Range X Scale", "[Axis] Range Y Scale", "[Layout] Graph Type Change", "[Plot] Tacho Point", "[Plot] Grid and BG", "[Cursor] Cursor Info", "[Legend] Pair Strings", "[Data] Plot Data", "[Legend] Checkbox", "[Layout] Update", "[Legend] Tree Open", "[Layout] Legend Visible Change", "[Plot] Data Point", "[Cursor] Appearance", "[Cursor] Index", "[Legend] Color", "[Axis] Axis and Label", "[Axis] Format String", "[Layout] Min Pane Size", "[Data] Index", "[Plot] Caption", "[Data] Legend Strings"] ("f")
        n419 = event-data() -> ("Tag"=w951:string)  [unwired: 1 in]
        n420 = Unbundle By Name(w945) -> ("Data Related State"=w949:T6)
        n421 = Dequeue Element(queue=w949) -> (queue out=w946:T6, element=w944:T13)  [unwired: 2 in, 2 out]
        n422 = Unbundle By Name(w944) -> ("Parents Tags"=w948:string[], "Open?"=w947:bool[])
        n423 = Search 1D Array(1D array=w948, element=w951) -> (index of element=w955:i32)  [unwired: 1 in]
        n424 = Index Array(array=w947, index=w955) -> (element=w952:bool)
        n425 = Bundle By Name(cluster=w957, "State Changed?"=TRUE, "Action Name"="Item Open") -> (w956:T2)
        n426 = Not(x=w952) -> (.not. x?=w953:bool)
        n427 = Replace Array Subset(array=w947, new element=w953, index=w955) -> (w954:bool[])
        n428 = Bundle By Name(cluster=w944, "Open?"=w954) -> (w943:T13)
        n429 = Enqueue Element(queue=w946, element=w943) -> ()  [unwired: 2 in, 3 out]
      }
      event "Tree": Mouse Down {
        n430 = event-data() -> ("Coords"=w969:T1)  [unwired: 1 in]
        n431 = Unbundle By Name(w973) -> ("Data Related State"=w966:T6, "Legend Background"=w968:u32)
        n432 = Dequeue Element(queue=w966) -> (queue out=w962:T6, element=w960:T13)  [unwired: 2 in, 2 out]
        n433 = Unbundle By Name(w960) -> ("Parents Tags"=w965:string[], "Children Tags"=w964:string[])
        n434 = control-ref of="Tree"() -> (w977:refnum<vi>)
        n435 = call <vilib>:"svx_Timebase CheckboxToIndex.vi"("All Children Tags"=w964, "All parents Tags"=w965, "Coords"=w969, "Tree ref in"=w977) -> ("State Changed?"=w976:bool, "index"=w975:cluster{"RowIdx":i32, "ColumnIdx":i32}[])  [unwired: 5 in, 1 out]
        n436 = case shown="False" w976 {
          tunnel: w973 -> [w985 w1007]
          tunnel: w975 -> [_ w997]
          tunnel: [w984 w1006] -> w972
          tunnel: w971 -> [w981 w1003]
          tunnel: [w980 w1002] -> w970
          tunnel: w968 -> [w986 _]
          tunnel: [_ w1001] -> w967
          tunnel: [w979 w1000] -> w963
          tunnel: w962 -> [w979 w1000]
          tunnel: [w978 w998] -> w961
          tunnel: w960 -> [w978 w999]
          frame False {
            w987 = -2 ("Active Cell:Active Column Number")
            n437 = property on="Tree" class="Tree (strict)"("ActiveColNum"=w987, "Active Item Row Number"=w987) -> ("CellBG"=w983:u32)  [unwired: 2 in, 2 out]
            n438 = Equal?(x=w983, y=w986) -> (x = y?=w982:bool)
            n439 = case shown="False" w982 {
              tunnel: w985 -> [w992 w996]
              tunnel: [w991 w996] -> w984
              tunnel: [w990 w995] -> w980
              tunnel: w983 -> [w989 _]
              tunnel: w981 -> [w988 w995]
              frame False {
                n440 = Bundle By Name(cluster=w988, "State Changed?"=TRUE, "Action Name"="Color Change") -> (w990:T2)
                n441 = Bundle By Name(cluster=w992, "Legend Background"=w989) -> (w991:T3)
              }
              frame True {
              }
            }
          }
          frame True {
            w1001 = T12[] [enum."[Data] Plot Data", enum."[Axis] Range X Scale", enum."[Axis] Range Y Scale", enum."[Cursor] Index", enum."[Cursor] Cursor Info"] items=["None", "[Axis] Range X Scale", "[Axis] Range Y Scale", "[Layout] Graph Type Change", "[Plot] Tacho Point", "[Plot] Grid and BG", "[Cursor] Cursor Info", "[Legend] Pair Strings", "[Data] Plot Data", "[Legend] Checkbox", "[Layout] Update", "[Legend] Tree Open", "[Layout] Legend Visible Change", "[Plot] Data Point", "[Cursor] Appearance", "[Cursor] Index", "[Legend] Color", "[Axis] Axis and Label", "[Axis] Format String", "[Layout] Min Pane Size", "[Data] Index", "[Plot] Caption", "[Data] Legend Strings"]
            n442 = Bundle By Name(cluster=w1007, "Index"=w997) -> (w1006:T3)
            n443 = Bundle By Name(cluster=w1003, "State Changed?"=TRUE, "Action Name"="Selector Changed") -> (w1002:T2)
            n444 = Bundle By Name(cluster=w999, "Index"=w997) -> (w998:T13)
          }
        }
        n445 = Enqueue Element(queue=w963, element=w961) -> ()  [unwired: 2 in, 3 out]
      }
      event "Split": Mouse Enter {
        n446 = event-data() -> ()  [unwired: 1 in, 1 out]
        n447 = Unbundle By Name(w1014) -> ("Refnum"=w1013:refnum<vi>)
        n448 = property class="Ctl"(reference=w1013) -> ("OwningVI"=w1009:refnum<vi>)  [unwired: 1 in, 2 out]
        n449 = Unbundle By Name(w1010) -> ("Cursor ID"=w1008:refnum<k1>)
        n450 = call-poly <vilib>:"Set Cursor.vi"("VI reference (current VI)"=w1009, "cursor ID"=w1008) -> ()  [unwired: 8 in, 2 out]
      }
      event "Split": Mouse Down {
        w1016 = cluster{u32, u32} {16777216, 16777216}
        # "Do not allow users to colorize the split."
        n451 = event-data() -> ("CtlRef"=w1017:refnum<vi>, "Coords.Horizontal"=→"Orig Coord":i32)  [unwired: 1 in]
        n452 = Build Array(w1016, w1016, w1016, w1016) -> (w1015:cluster{u32, u32}[])
        n453 = property class="Bool (strict)"(reference=w1017, "Colors [4]"=w1015) -> ()  [unwired: 1 in, 2 out]
      }
      event Mouse Move {
        n454 = event-data() -> ("Coords.Horizontal"=w1026:i32)  [unwired: 1 in]
        n455 = local read "Split"() -> (w1027:bool)
        n456 = case shown="True" w1027 {
          tunnel: w1026 -> [_ w1051]
          tunnel: w1025 -> [_ w1049]
          tunnel: w1022 -> [_ w1037]
          frame False {
          }
          frame True {
            n457 = Unbundle By Name(w1049) -> ("Data Related State"=w1033:T6, "Legend Width"=w1048:u32, "Cursor ID"=w1036:refnum<k1>)
            n458 = Unbundle By Name(w1037) -> ("Refnum"=w1038:refnum<vi>)
            n459 = property class="Ctl"(reference=w1038) -> ("OwningVI"=w1039:refnum<vi>)  [unwired: 1 in, 2 out]
            n460 = Preview Queue Element(queue=w1033) -> (element=w1031:T13)  [unwired: 2 in, 3 out]
            n461 = call-poly <vilib>:"Set Cursor.vi"("VI reference (current VI)"=w1039, "cursor ID"=w1036) -> ()  [unwired: 8 in, 2 out]
            n462 = Unbundle By Name(w1031) -> ("Container Bounds.Width"=w1030:u32, "Tree Item Width"=w1032:u32)
            n463 = local read "Orig Coord"() -> (w1050:i32)
            n464 = Subtract(x=w1051, y=w1050) -> (x-y=w1047:i32)
            n465 = To Long Integer(number=w1048) -> (32bit integer=w1035:i32)
            n466 = To Long Integer(number=w1030) -> (32bit integer=w1034:i32)
            n467 = Subtract(x=w1035, y=w1047) -> (x-y=w1045:i32)
            n468 = Subtract(x=w1034, y=20) -> (x-y=w1029:i32)
            n469 = Subtract(x=w1029, y=w1045) -> (x-y=w1040:i32)
            n470 = Greater Or Equal?(x=w1045, y=100) -> (x >= y?=w1042:bool)
            n471 = Greater Or Equal?(x=w1040, y=150) -> (x >= y?=w1043:bool)
            n472 = And(x=w1043, y=w1042) -> (x .and. y?=w1041:bool)
            n473 = case shown="True" w1041 {
              tunnel: w1045 -> [_ w1054]
              tunnel: w1040 -> [_ w1057]
              tunnel: w1032 -> [_ w1056]
              frame False {
              }
              frame True {
                n474 = Subtract(x=w1057, y=106) -> (x-y=w1062:i32)
                n475 = property on="Probe X" class="XYGraph (strict)"("Width"=w1062) -> ("Width"=w1060:u32, "Left"=w1059:i32)  [unwired: 2 in, 2 out]
                n476 = property on="Probe Y" class="XYGraph (strict)"("Width"=w1062) -> ()  [unwired: 2 in, 2 out]
                n477 = Add(x=w1060, y=w1059) -> (x+y=w1058:u32)
                n478 = Subtract(x=w1054, y=u32 25) -> (x-y=w1053:u32)
                n479 = Max & Min(x=w1056, y=w1053) -> (max(x,y)=w1052:u32)  [unwired: 1 out]
                n480 = property on="Tree" class="Tree (strict)"("Width"=w1052, "Width"=w1054, "Left"=w1058) -> ()  [unwired: 2 in, 2 out]
                n481 = property on="Split" class="Bool (strict)"("Left"=w1058) -> ()  [unwired: 2 in, 2 out]
              }
            }
          }
        }
      }
      event Mouse Leave {
        n482 = event-data() -> ()  [unwired: 1 in, 1 out]
        n483 = local read "Split"() -> (w1068:bool)
        n484 = case shown="True" w1068 {
          tunnel: w1070 -> [w1073 w1085]
          tunnel: [w1073 w1084] -> w1067
          tunnel: w1066 -> [w1072 w1081]
          tunnel: [w1072 w1080] -> w1065
          tunnel: w1064 -> [_ w1076]
          tunnel: [w1071 w1074] -> w1063
          frame False {
            w1071 = T12[] [] items=["None", "[Axis] Range X Scale", "[Axis] Range Y Scale", "[Layout] Graph Type Change", "[Plot] Tacho Point", "[Plot] Grid and BG", "[Cursor] Cursor Info", "[Legend] Pair Strings", "[Data] Plot Data", "[Legend] Checkbox", "[Layout] Update", "[Legend] Tree Open", "[Layout] Legend Visible Change", "[Plot] Data Point", "[Cursor] Appearance", "[Cursor] Index", "[Legend] Color", "[Axis] Axis and Label", "[Axis] Format String", "[Layout] Min Pane Size", "[Data] Index", "[Plot] Caption", "[Data] Legend Strings"] ("f")
          }
          frame True {
            w1074 = T12[] [enum."[Layout] Min Pane Size"] items=["None", "[Axis] Range X Scale", "[Axis] Range Y Scale", "[Layout] Graph Type Change", "[Plot] Tacho Point", "[Plot] Grid and BG", "[Cursor] Cursor Info", "[Legend] Pair Strings", "[Data] Plot Data", "[Legend] Checkbox", "[Layout] Update", "[Legend] Tree Open", "[Layout] Legend Visible Change", "[Plot] Data Point", "[Cursor] Appearance", "[Cursor] Index", "[Legend] Color", "[Axis] Axis and Label", "[Axis] Format String", "[Layout] Min Pane Size", "[Data] Index", "[Plot] Caption", "[Data] Legend Strings"] ("f")
            n485 = Unbundle By Name(w1076) -> ("Refnum"=w1078:refnum<vi>)
            n486 = Unbundle By Name(w1085) -> ("Legend Width"=→"Orig Legend Width":u32)
            n487 = property class="Ctl"(reference=w1078) -> ("OwningVI"=w1077:refnum<vi>)  [unwired: 1 in, 2 out]
            n488 = call-poly <vilib>:"Set Cursor.vi"("VI reference (current VI)"=w1077, "icon"=u16 0) -> ()  [unwired: 8 in, 2 out]
            n489 = property on="Tree" class="Tree (strict)"() -> ("Width"=w1079:u32)  [unwired: 2 in, 2 out]
            n490 = Bundle By Name(cluster=w1085, "Legend Width"=w1079) -> (w1084:T3)
            n491 = Bundle By Name(cluster=w1081, "Action Name"="Resize", "State Changed?"=TRUE) -> (w1080:T2)
          }
        }
      }
      event Mouse Enter {
        n492 = event-data() -> ()  [unwired: 1 in, 1 out]
        n493 = local read "Split"() -> (w1091:bool)
        n494 = case shown="True" w1091 {
          tunnel: w1093 -> [w1095 w1097]
          tunnel: [w1095 w1106] -> w1090
          tunnel: w1089 -> [w1094 w1102]
          tunnel: [w1094 w1101] -> w1088
          tunnel: w1087 -> [_ w1098]
          frame False {
          }
          frame True {
            n495 = Unbundle By Name(w1098) -> ("Refnum"=w1099:refnum<vi>)
            n496 = Unbundle By Name(w1097) -> ("Cursor ID"=w1096:refnum<k1>)
            n497 = property class="Ctl"(reference=w1099) -> ("OwningVI"=w1100:refnum<vi>)  [unwired: 1 in, 2 out]
            n498 = call-poly <vilib>:"Set Cursor.vi"("VI reference (current VI)"=w1100, "cursor ID"=w1096) -> ()  [unwired: 8 in, 2 out]
            n499 = local read "Orig Legend Width"() -> (w1105:u32)
            n500 = Bundle By Name(cluster=w1102, "Action Name"="Resize", "State Changed?"=TRUE) -> (w1101:T2)
            n501 = Bundle By Name(cluster=w1097, "Legend Width"=w1105) -> (w1106:T3)
          }
        }
      }
      event Mouse Up {
        n502 = event-data() -> ()  [unwired: 1 in, 1 out]
        n503 = Unbundle By Name(w1114) -> ("Legend Width"=w1109:u32)
        n504 = property on="Tree" class="Tree (strict)"() -> ("Width"=w1110:u32)  [unwired: 2 in, 2 out]
        n505 = Not Equal?(x=w1110, y=w1109) -> (x != y?=w1115:bool)
        n506 = case shown="True" w1115 {
          tunnel: w1114 -> [w1119 w1131]
          tunnel: w1110 -> [_ w1125]
          tunnel: [w1119 w1126] -> w1113
          tunnel: w1112 -> [w1118 w1128]
          tunnel: [w1118 w1127] -> w1111
          tunnel: w1108 -> [_ w1121]
          tunnel: [w1117 w1120] -> w1107
          frame False {
            w1117 = T12[] [] items=["None", "[Axis] Range X Scale", "[Axis] Range Y Scale", "[Layout] Graph Type Change", "[Plot] Tacho Point", "[Plot] Grid and BG", "[Cursor] Cursor Info", "[Legend] Pair Strings", "[Data] Plot Data", "[Legend] Checkbox", "[Layout] Update", "[Legend] Tree Open", "[Layout] Legend Visible Change", "[Plot] Data Point", "[Cursor] Appearance", "[Cursor] Index", "[Legend] Color", "[Axis] Axis and Label", "[Axis] Format String", "[Layout] Min Pane Size", "[Data] Index", "[Plot] Caption", "[Data] Legend Strings"] ("f")
          }
          frame True {
            w1120 = T12[] [enum."[Layout] Min Pane Size"] items=["None", "[Axis] Range X Scale", "[Axis] Range Y Scale", "[Layout] Graph Type Change", "[Plot] Tacho Point", "[Plot] Grid and BG", "[Cursor] Cursor Info", "[Legend] Pair Strings", "[Data] Plot Data", "[Legend] Checkbox", "[Layout] Update", "[Legend] Tree Open", "[Layout] Legend Visible Change", "[Plot] Data Point", "[Cursor] Appearance", "[Cursor] Index", "[Legend] Color", "[Axis] Axis and Label", "[Axis] Format String", "[Layout] Min Pane Size", "[Data] Index", "[Plot] Caption", "[Data] Legend Strings"] ("f")
            n507 = Unbundle By Name(w1121) -> ("Refnum"=w1122:refnum<vi>)
            n508 = Bundle By Name(cluster=w1131, "Legend Width"=w1125) -> (w1126:T3)
            n509 = property class="Ctl"(reference=w1122) -> ("OwningVI"=w1123:refnum<vi>)  [unwired: 1 in, 2 out]
            n510 = call-poly <vilib>:"Set Cursor.vi"("VI reference (current VI)"=w1123, "icon"=u16 0) -> ()  [unwired: 8 in, 2 out]
            n511 = Bundle By Name(cluster=w1128, "Action Name"="Resize", "State Changed?"=TRUE) -> (w1127:T2)
          }
        }
      }
      event "Split": Mouse Leave {
        n512 = event-data() -> ()  [unwired: 1 in, 1 out]
        n513 = Unbundle By Name(w1138) -> ("Refnum"=w1137:refnum<vi>)
        n514 = property class="Ctl"(reference=w1137) -> ("OwningVI"=w1136:refnum<vi>)  [unwired: 1 in, 2 out]
        n515 = call-poly <vilib>:"Set Cursor.vi"("VI reference (current VI)"=w1136, "icon"=u16 0) -> ()  [unwired: 8 in, 2 out]
      }
      event Mouse Down {
        n516 = event-data() -> ("Button"=w1139:u16, "Mods"=w1141:cluster{"Double Click":bool, "Menu Key":bool}, "Coords"=w1140:T1)  [unwired: 1 in]
        n517 = case shown="1" w1139 {
          tunnel: w1141 -> [w1150 _]
          tunnel: w1140 -> [w1149 _]
          frame 1 {
            n518 = local read "Coords"() -> (w1148:T1)
            n519 = Unbundle By Name(w1150) -> ("Double Click"=w1146:bool)
            n520 = Equal?(x=w1149, y=w1148) -> (x = y?=w1147:bool)
            n521 = And(x=w1146, y=w1147) -> (x .and. y?=w1145:bool)
            n522 = case shown="True" w1145 {
              frame False {
              }
              frame True {
                n523 = control-ref of="This VI"() -> (w1152:refnum<vi>)
                n524 = property class="FcdVI"(reference=w1152, "BDWin.Open"=FALSE ("Block Diagram Window:Open")) -> ()  [unwired: 1 in, 2 out]
              }
            }
          }
          frame 0, Default {
          }
        }
      }
    }
    n525 = Empty Array?(array=w9) -> (empty?=w10:bool)
    n526 = case shown="False" w10 {
      tunnel: w14 -> [w20 w26]
      tunnel: w13 -> [_ w36]
      tunnel: [w20 w21] -> w12
      tunnel: w9 -> [_ w35]
      tunnel: w8 -> [_ w22]
      frame True {
      }
      frame False {
        n527 = control-ref of="Probe X"() -> (w33:refnum<vi>)
        n528 = control-ref of="Probe Y"() -> (w32:refnum<vi>)
        n529 = control-ref of="Tree"() -> (w31:refnum<vi>)
        n530 = Unbundle By Name(w22) -> ("Refnum"=w23:refnum<vi>)
        n531 = control-ref of="Split"() -> (w30:refnum<vi>)
        n532 = control-ref of="cursor X info"() -> (w29:refnum<vi>)
        n533 = control-ref of="cursor Y info"() -> (w28:refnum<vi>)
        n534 = control-ref of="This VI"() -> (w34:refnum<vi>)
        n535 = Bundle("Probe X"=w33, "Probe Y"=w32, "Tree"=w31, "Split"=w30, "cursor X info"=w29, "cursor Y info"=w28) -> (w27:T16)  [unwired: 1 in]
        n536 = call <vilib>:"svx_Timebase Queue To State.vi"("Display State In"=w26) -> ("Display State Out"=w25:T3)  [unwired: 10 in]
        n537 = call <vilib>:"svx_Timebase Exec Commands.vi"("Display State In"=w25, "Data In"=w36, "Commands"=w35, "Facade VI"=w34, "Ref Ins"=w27, "Container"=w23) -> ("Display State Out"=w24:T3)  [unwired: 5 in]
        n538 = call <vilib>:"svx_Timebase State To Queue.vi"("Display State In"=w24) -> ("Display State Out"=w21:T3)  [unwired: 10 in]
      }
    }
  }
  "Display State Out" <- w4
  "Data Out" <- w7
  "Action" <- w2
